vi "4Pi Objective Lock - EMBL.vi"(7 "Calling VI Ref":refnum<vi>) -> ()   [LabVIEW 2016]
uses:
  <vilib>/Utility/miscctls.llb/LVPointTypeDef.ctl
  4Pi Objective Lock Type Defs/4Pi Obj Lock - Notifier Type.ctl
  4Pi Objective Lock Type Defs/4Pi Obj Lock - Actions.ctl
  <vilib>/vision/Image Controls.llb/IMAQ Image.ctl
  4Pi Objective Lock Type Defs/4Pi Obj Lock - Lock Settings.ctl
  Hardware Configuration/Hardware Configuration Controls/Device Type.ctl
  Hardware Configuration/Hardware Configuration Controls/Device Function.ctl
  4Pi Objective Lock Type Defs/4Pi Obj Lock - Camera Settings.ctl
  Device Library/Cameras/Camera Controls/Generic Camera ROI.ctl
  Device Library/Cameras/Camera Controls/Generic Camera Actions.ctl
  Device Library/Stages/Stages Controls/Stage Actions.ctl
  <vilib>/addons/control/pid/pid.llb/PID (DBL Array).vi
  <vilib>/addons/control/pid/pid.llb/PID (DBL).vi
  <vilib>/addons/control/pid/NI_PID_pid.lvlib
  <vilib>/vision/NI_Vision_Development_Module.lvlib
panel:
  out "dxy (px)":dbl[](array[numeric])
  out "dz (µm)":dbl format="%.2f"
  in  "Main Tab":T1(tab)
  out "Z Move":bool
  out "XY Move":bool
  out "Measured X Position (px)":dbl=1.0 format="%.3g"
  out "Measured Y Position (px)":dbl=1.0 format="%.3g"
  out "Measured sx/sy":dbl=1.0 format="%.3g"
  out "Target X Position (px)":dbl=1.0 format="%.3g"
  out "Target Y Position (px)":dbl=1.0 format="%.3g"
  out "Target sx/sy":dbl=1.0 format="%.3g"
  out "Z Axis Position (µm)":dbl=1.0 format="%.4g"
  out "Y Axis Position (µm)":dbl=1.0 format="%.2g"
  out "X Axis Position (µm)":dbl=1.0 format="%.2g"
  out "Z Target and Fit Value (µm)":T2(graph)
  in  "Start Lock":bool
  out "Y Target and Fit Position (µm)":T2(graph)
  out "X Target and Fit Position (µm)":T2(graph)
  in  "Restart Lock":bool
  out "Fit Error":bool
  out "Move Limit Error":bool
  out "Target Z (µm)":dbl=1.0 format="%.3g"
  out "Measured Z (µm)":dbl=1.0 format="%.3g"
  out "Target X Position cc (px)":dbl=1.0 format="%.3g"
  out "Measured X Position cc (px)":dbl=1.0 format="%.3g"
  out "Measured Y Position cc (px)":dbl=1.0 format="%.3g"
  out "Target Y Position cc (px)":dbl=1.0 format="%.3g"
  in  "pixel size (µm)":dbl=0.01
  in  "X Update Scale Factor":dbl=0.01
  in  "Y Update Scale Factor":dbl=0.01
  in  "Z Update Scale Factor":dbl=0.2
  in  "Sample Z Step No.":u32=2
  in  "Sample Z Step Size (µm)":dbl=2.0
  in  "Update Delay (ms)":i32=10
  in  "D (Derivative)":dbl
  in  "I (Integral)":dbl
  in  "P (Proportional)":dbl=2.0
  in  "Invert Z Axis":bool
  in  "XY Drift Threshold":dbl=0.05
  in  "Abort If Error":bool
  in  "Flip XY Axis":bool
  in  "Invert X Axis":bool=TRUE
  in  "Invert Y Axis":bool=TRUE
  in  "Z Stage Move Limit (µm)":dbl=5.0
  in  "Z Drift Threshold":dbl=0.05
  in  "XY Stage Move Limit (µm)":dbl=1.0
  in  "Frame Accumulations":u16=10
  in  "XY Correction Active":bool=TRUE
  in  "Z Correction Active":bool=TRUE
  in  "Set Camera ROI":bool
  in  "Save Lock Settings":bool
  in  "Quit":bool
  # "Z Drift Settings"
  # "Camera Setup"
  # "XY Drift Settings"
  # "PID Control Values"
  # "General Settings"
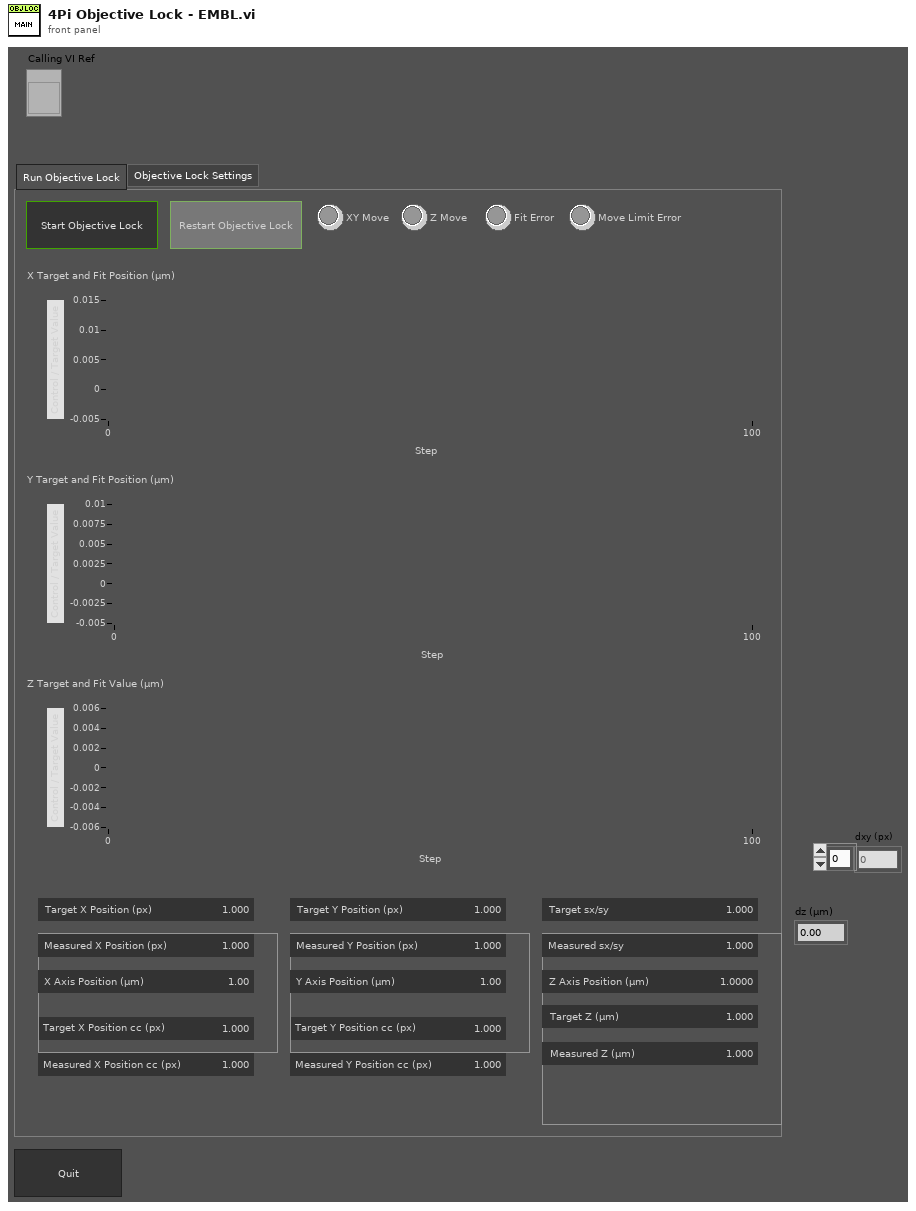
[diagram p1: front panel]
types:
  T1 = enum32{"Run Objective Lock", "Objective Lock Settings"}
  T2 = cluster{"Target 01":dbl, dbl, dbl, "Current 01":dbl, "Stage Pos":dbl}
  T3 = typedef "4Pi Obj Lock - Camera Settings.ctl" = cluster{"Exposure Time (s)":dbl, "H Offset":u16, "V Offset":u16, "H Width":u16, "V Width":u16}
  T4 = typedef "Device Function.ctl" = enum16{"Primary", "Secondary", "Overview", "Wide Field Drift Correction", "642 nm Excitation", "560 nm Excitation", "940 nm Excitation", "546 nm Excitation", "488 nm Excitation", "405 nm Excitation", "Objective Drift Correction", "4Pi Focus Lock", "4Pi Objective Lock", "Objective XY", "Objective Z", "Sample XY", "Sample Coarse Z", "Sample Z", "4Pi Lower", "4Pi Upper", "Mojo", "Adj Cavity", "Line Scanning", "Alert"}
  T5 = typedef "Device Type.ctl" = enum16{"AOTF", "Camera", "Deformable Mirror", "Laser", "Shutter", "Stage", "Waveform", "FPGA", "Email"}
  T6 = typedef "4Pi Obj Lock - Actions.ctl" = enum16{"Idle", "Start Lock", "Restart Lock", "Get Initial Position", "Get Target Z Position", "Get Ref Stack", "Cal Ref FFT", "Move To Init Z", "Get Current Z Position", "Get Current XY Position", "Get Current Position", "Check Drift", "Check Drift cc", "Move XYZ", "Move XY", "Move Z", "Update Plots", "Delay", "Abort", "Exit Loop", "Quit"}
  T7 = typedef "4Pi Obj Lock - Lock Settings.ctl" = cluster{"Z Drift Threshold":dbl, "Z Stage Move Limit (µm)":dbl, "XY Drift Threshold":dbl, "XY Stage Move Limit (µm)":dbl, "Frame Accumulations":u16, "Abort If Error":bool, "Flip XY Axis":bool, "Invert X Axis":bool, "Invert Y Axis":bool, "Invert Z Axis":bool, "Z Correction Active":bool, "XY Correction Active":bool, "PID Values":dbl[], "Update Delay (ms)":i32, "Sample Z Step Size (µm)":dbl, "Sample Z Step No.":u32, "Z Update Scale Factor":dbl, "Y Update Scale Factor":dbl, "X Update Scale Factor":dbl}
  T8 = typedef "4Pi Obj Lock - Notifier Type.ctl" = cluster{"Actions":T6, "Z Drift Threshold":dbl, "Z Stage Move Limit (µm)":dbl, "XY Drift Threshold":dbl, "XY Stage Move Limit (µm)":dbl, "Frame Accumulations":u16, "Abort If Error":bool, "Z Correction Active":bool, "XY Correction Active":bool, "PID Values":dbl[], "Running?":bool, "Update Delay (ms)":i32, "Cur Image (SGL)":T9, "Ref Stack (SGL)":T9[], "Sample Z (µm)":dbl[], "Initial Z Position (µm)":dbl, "Z Step Size (µm)":dbl, "Z Step No.":u32, "Ref FFT Stack (CSG)":T9[], "CC Image (SGL) ":T9, "Tmp Image FFT (CSG)":T9[], "CC Image Max (SGL)":T9}
  T9 = typedef "IMAQ Image.ctl" = refnum<image>
  T10 = enum16{"Always On", "Always Off", "Off While Running"}
  T11 = typedef "LVPointTypeDef.ctl" = cluster{"Horizontal":i16, "Vertical":i16}
  T12 = typedef "Image Type" = u32
  T13 = typedef "Generic Camera Actions.ctl" = enum16{"Status", "Live Preview", "Capture", "Abort", "Set Exposure Time (s)", "Get Exposure Time (s)", "Record Settings", "Set ROI", "Get ROI", "Defect Correction On/Off", "Cooler On/Off", "Fan On/Off", "Quit"}
  T14 = typedef "Generic Camera ROI.ctl" = cluster{"H_Offset":u16, "V_Offset":u16, "H_Width":u16, "V_Width":u16}
  T15 = typedef "Stage Actions.ctl" = enum16{"Get Position", "MVR", "MOVE", "HALT", "ONTARGET", "ERROR", "REFERENCE", "INIT", "VELOCITY", "STATUS", "EXIT", "HOME", "ZEROPOS", "NANOPOS", "ANALOG", "QUIT"}
  T16 = enum32{"Invalid", "Standard", "Closed", "Hidden", "Minimized", "Maximized"}
  T17 = cluster{"Target 01":dbl, dbl, dbl, "Current 01":dbl, "Stage Pos":dbl}[]
  T18 = typedef "Stage Status.ctl" = enum16{"Error", "Abort", "Busy", "On Target"}
  T19 = typedef "2D Gaussian - Best Fit Parameters.ctl" = cluster{"Amplitude":dbl, "X Position":dbl, "Y Position":dbl, "X Width":dbl, "Y Width":dbl, "Offset":dbl}
  T20 = cluster{"PID Values[0]":dbl, "PID Values[1]":dbl, "PID Values[2]":dbl}
  T21 = cluster{"PID Values[0]":dbl, "PID Values[1]":dbl, "PID Values[2]":dbl}[]
  T22 = typedef "LVRectTypeDef.ctl" = cluster{"Left":i16, "Top":i16, "Right":i16, "Bottom":i16}
  T23 = typedef "LVBoundsTypeDef.ctl" = cluster{"Width":u32, "Height":u32}
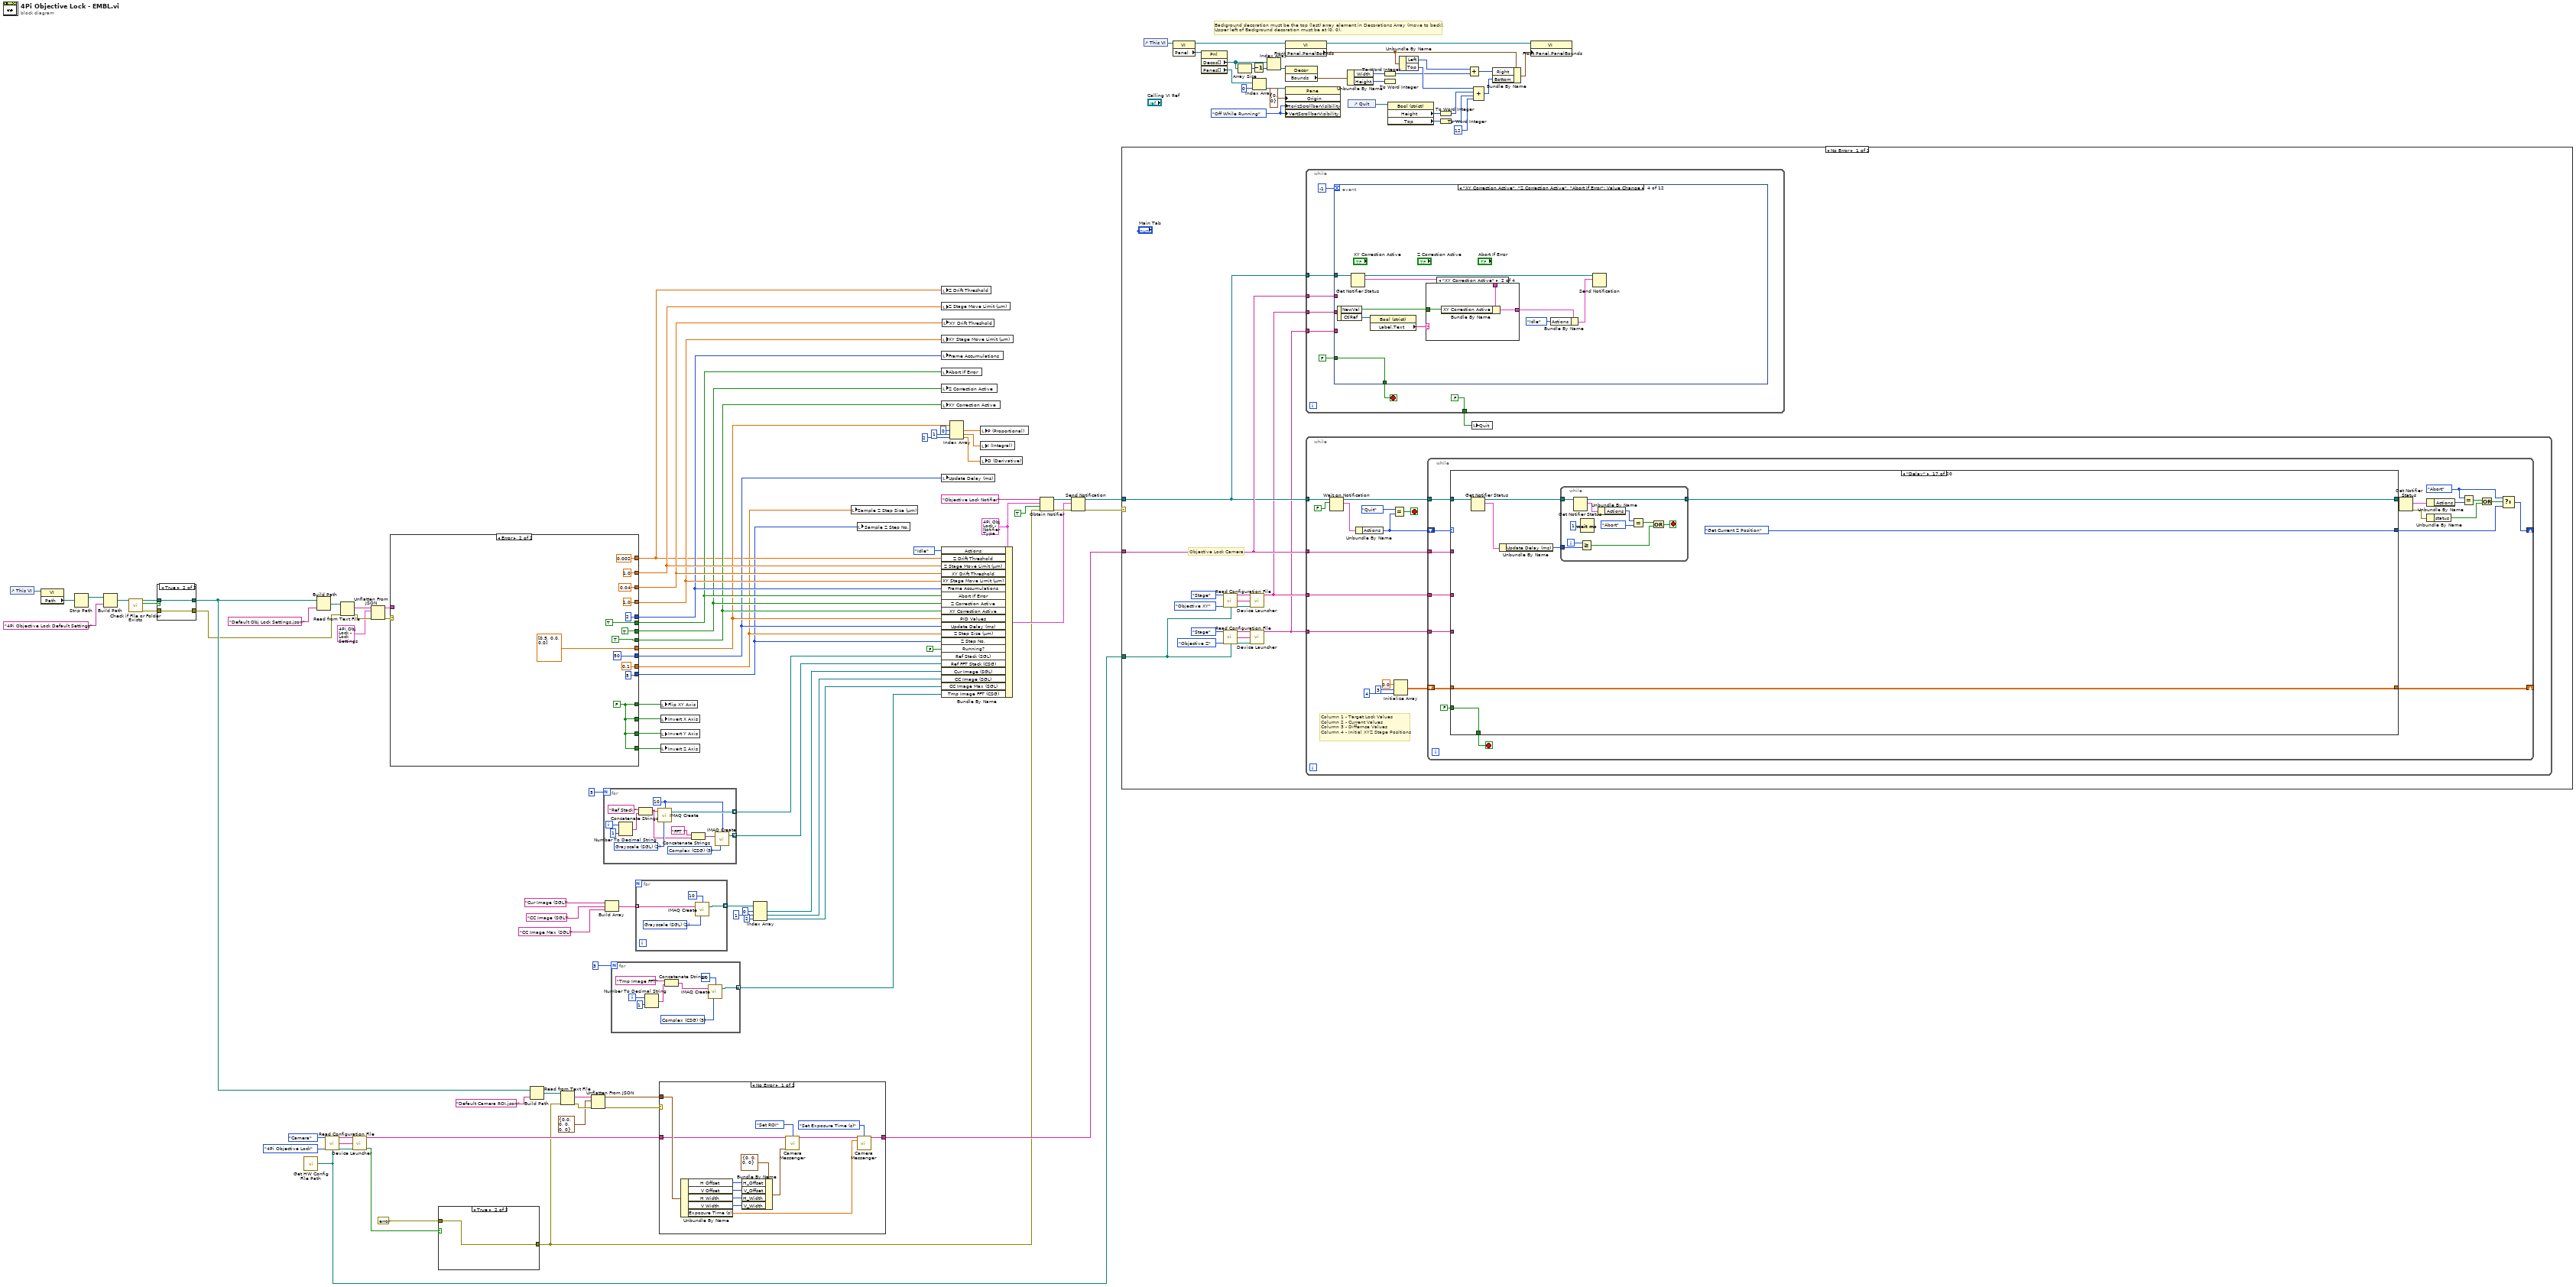
[diagram p0: block diagram]
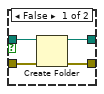
[diagram p2: hidden frame]
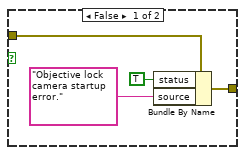
[diagram p3: hidden frame]
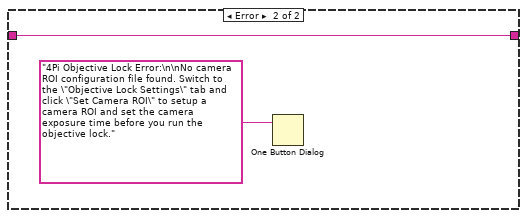
[diagram p4: hidden frame]
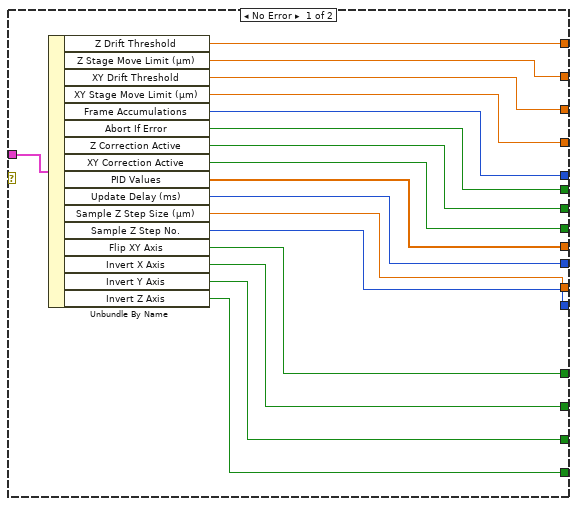
[diagram p5: hidden frame]
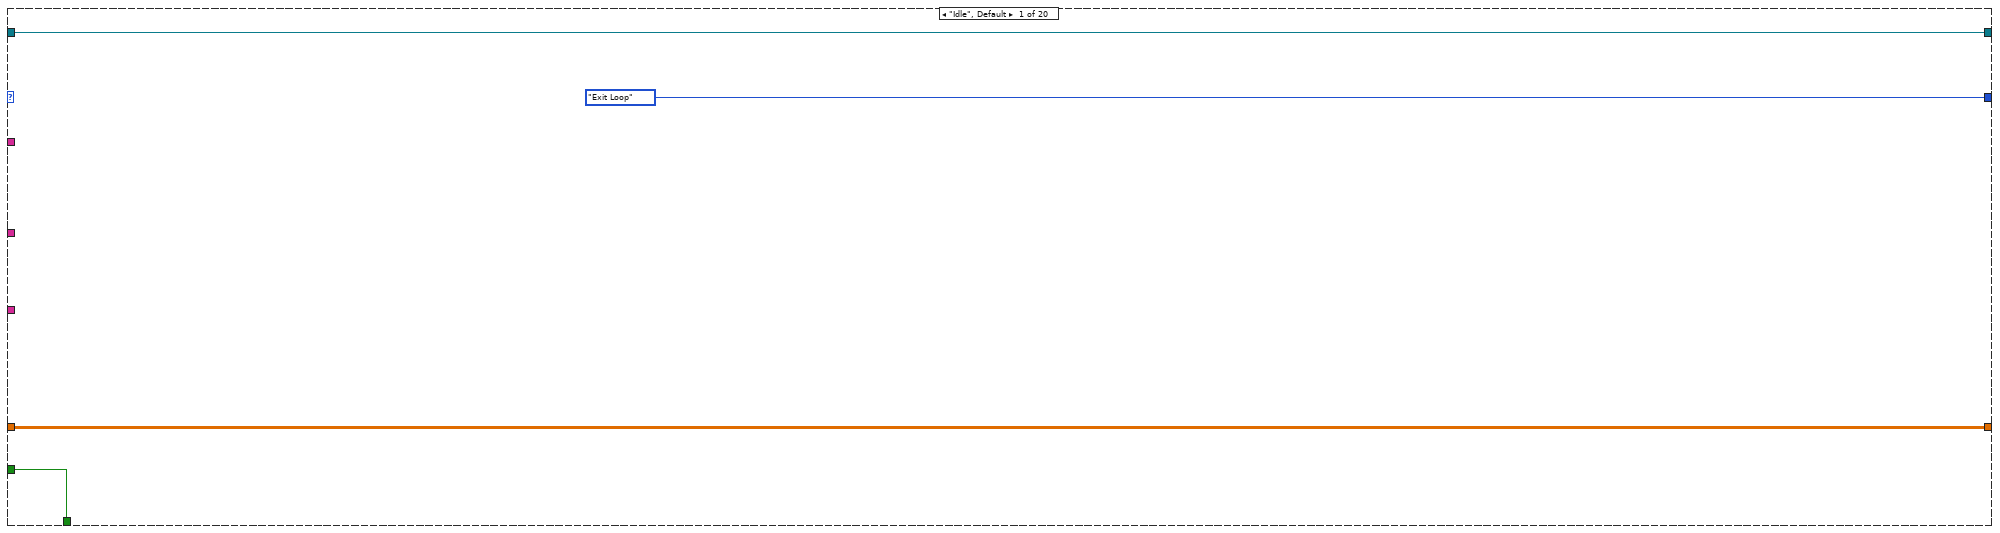
[diagram p6: hidden frame]
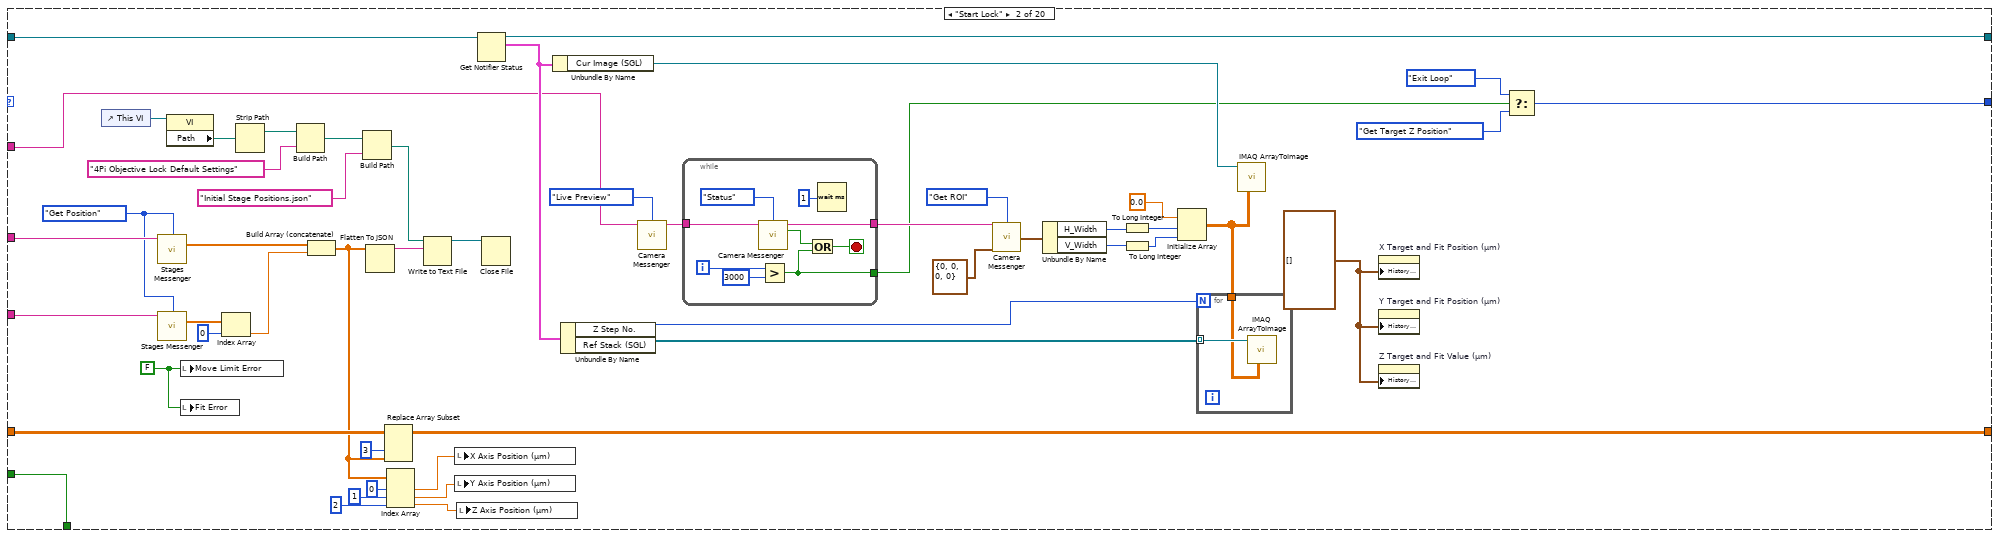
[diagram p7: hidden frame]
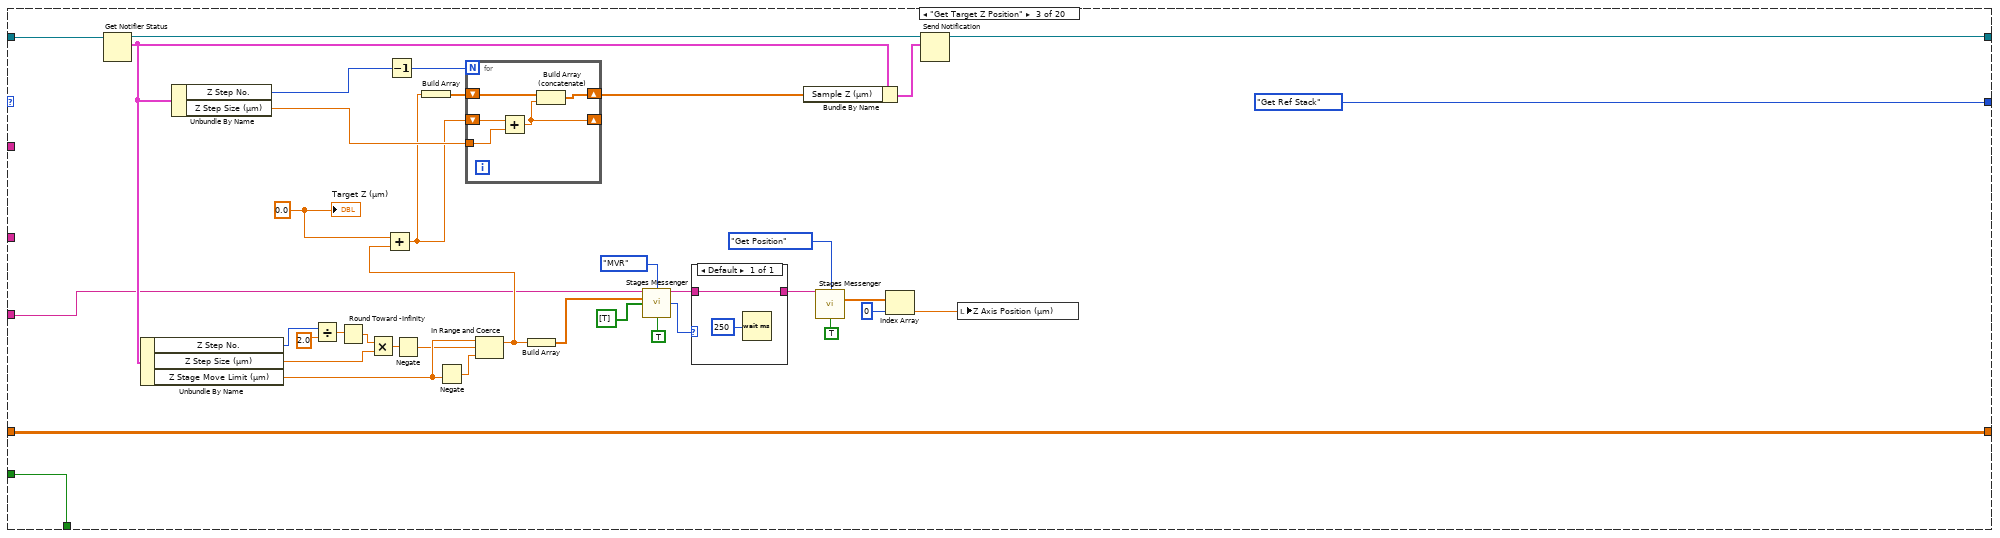
[diagram p8: hidden frame]
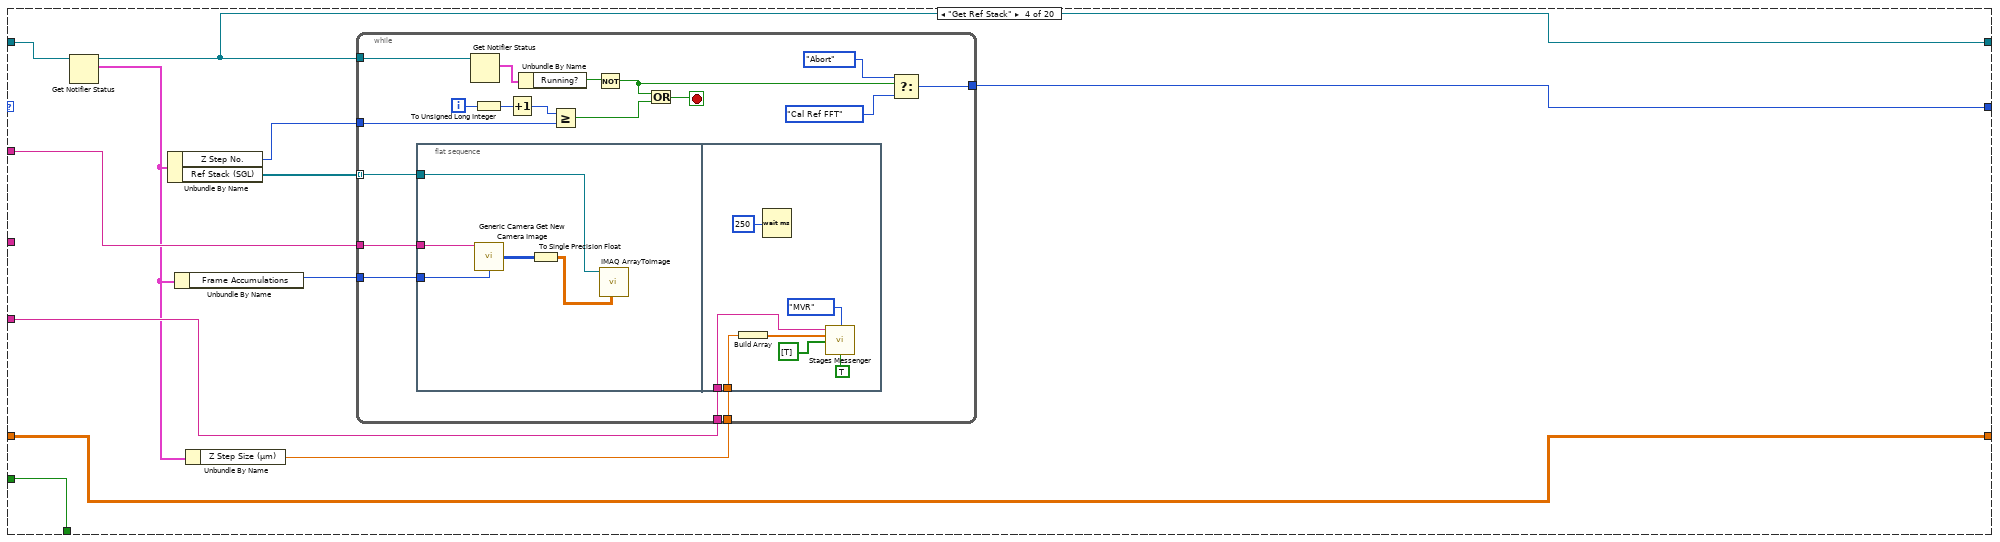
[diagram p9: hidden frame]
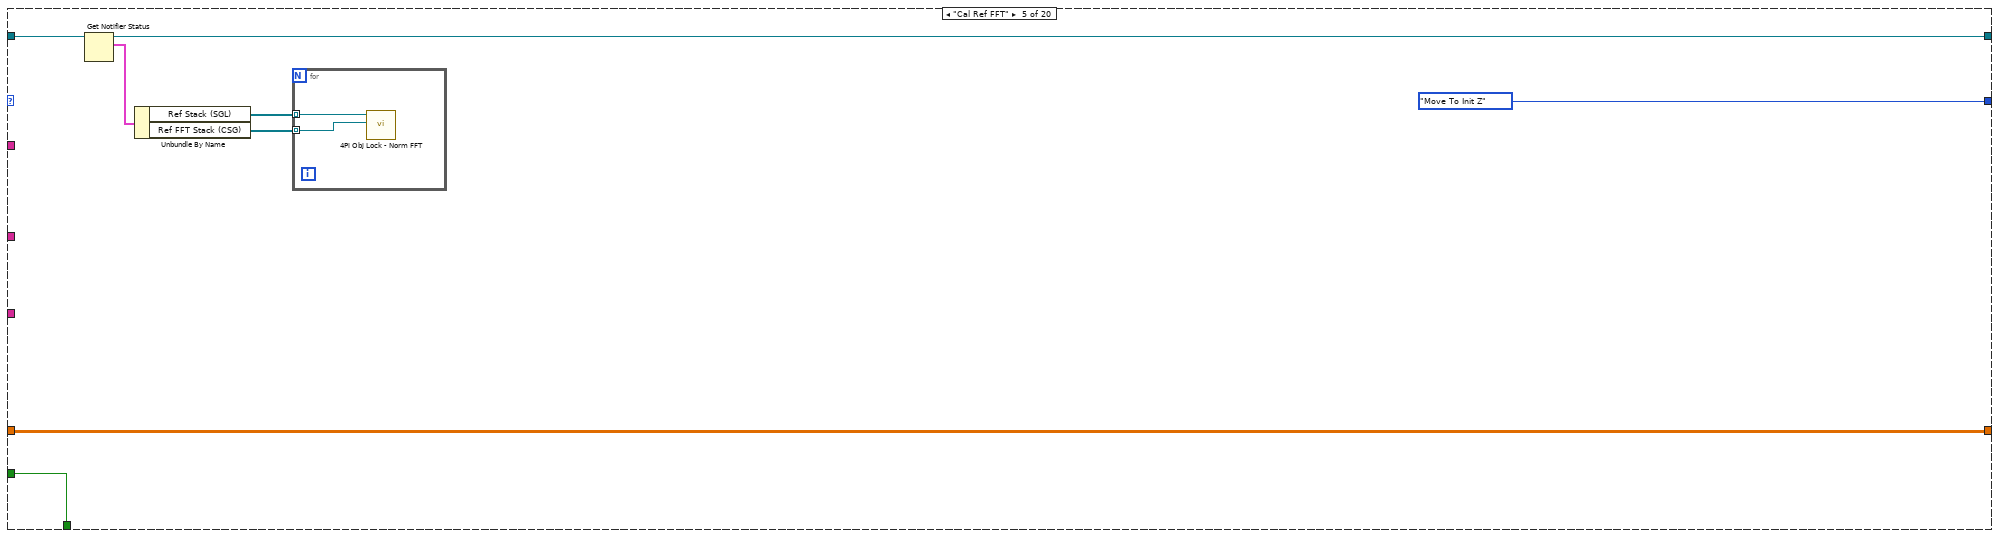
[diagram p10: hidden frame]
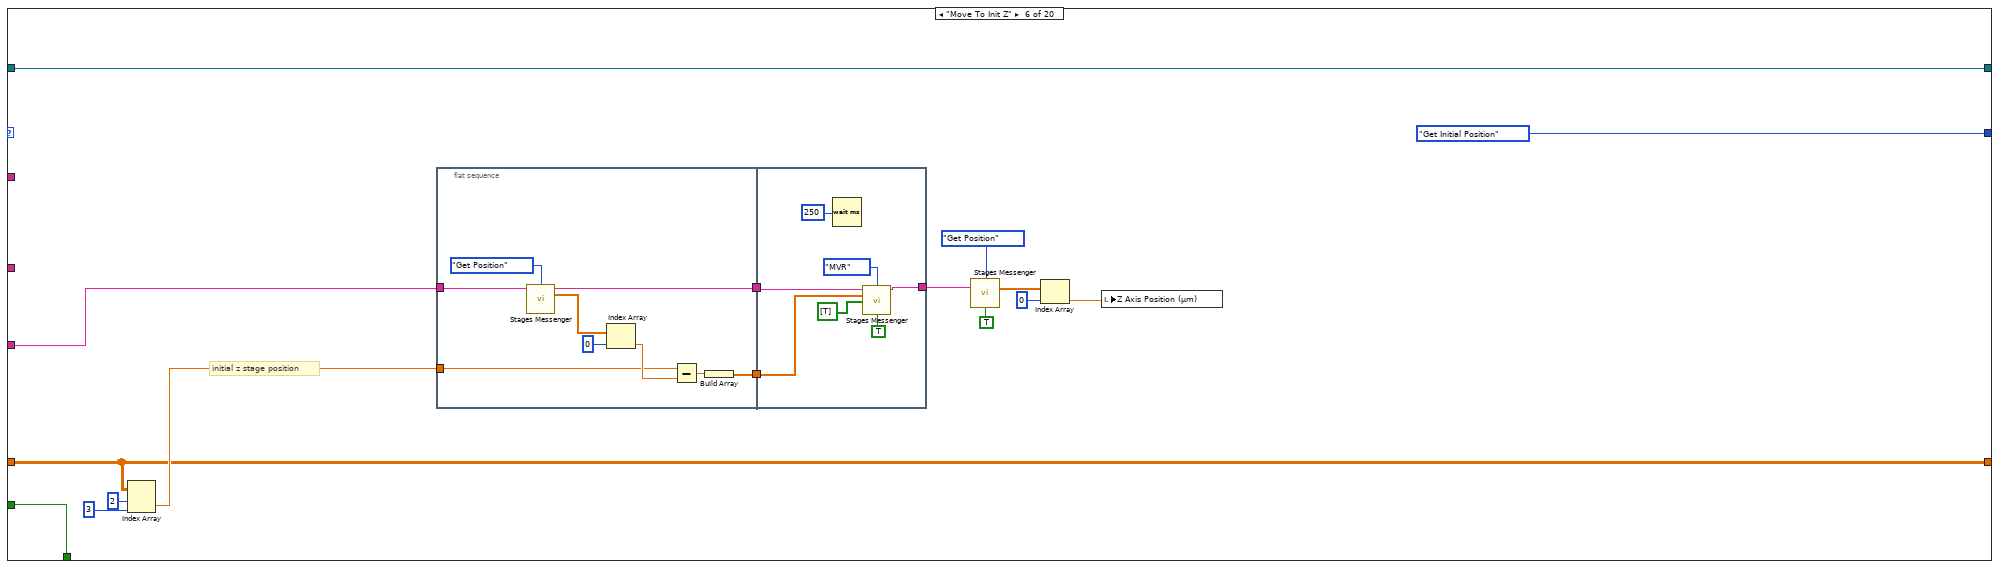
[diagram p11: hidden frame]
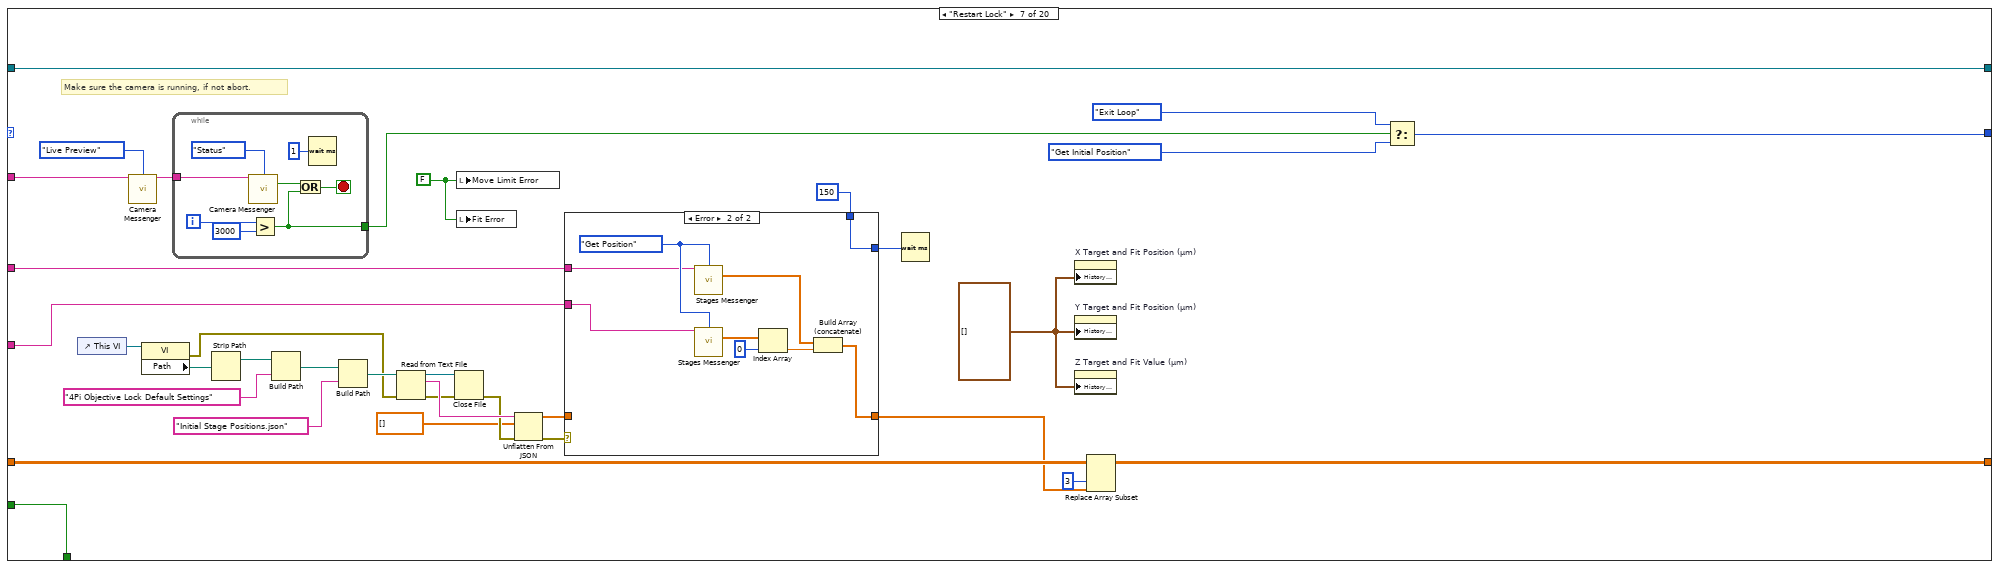
[diagram p12: hidden frame]
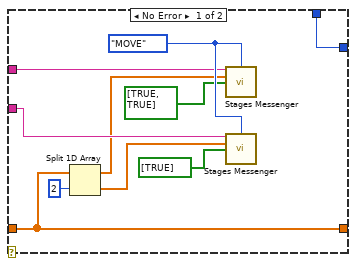
[diagram p13: hidden frame]
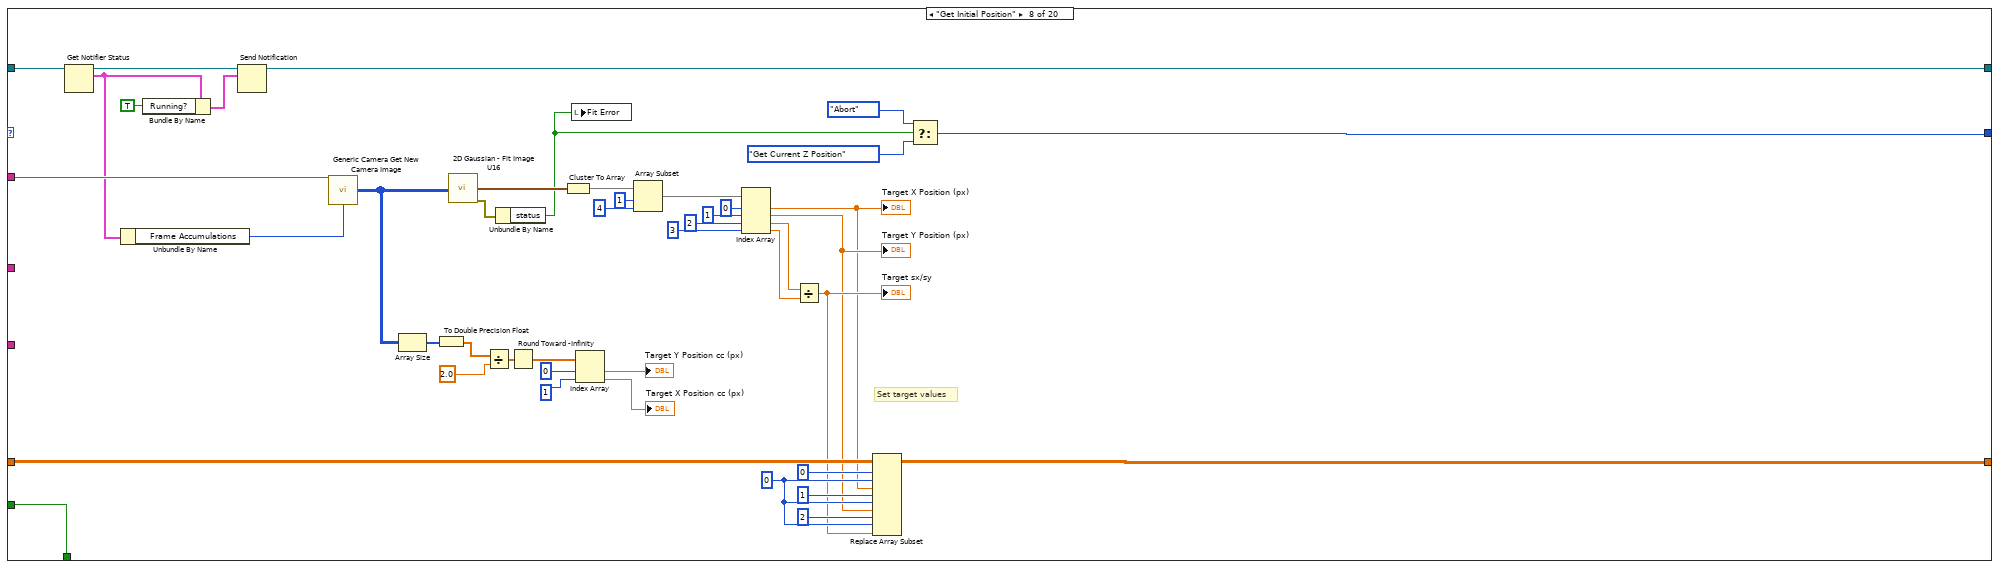
[diagram p14: hidden frame]
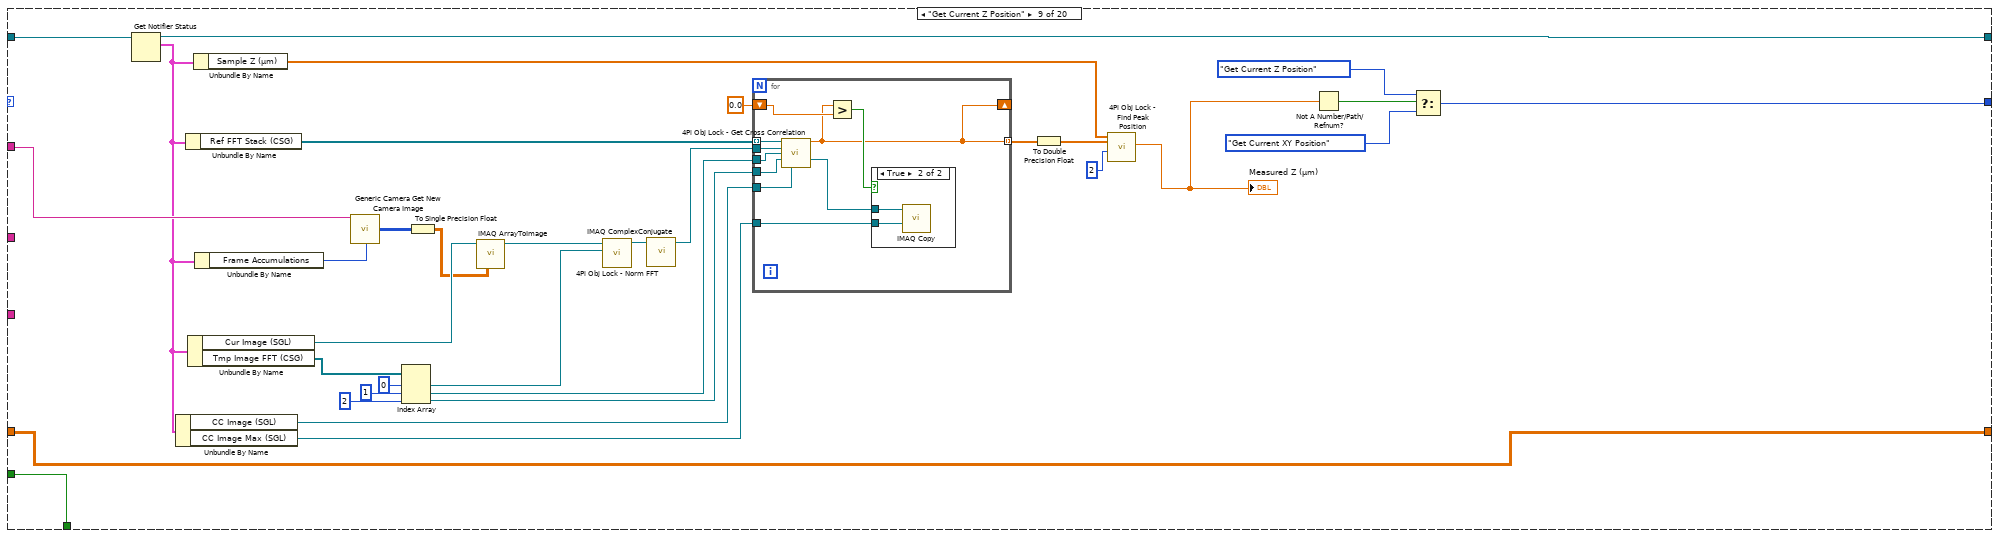
[diagram p15: hidden frame]
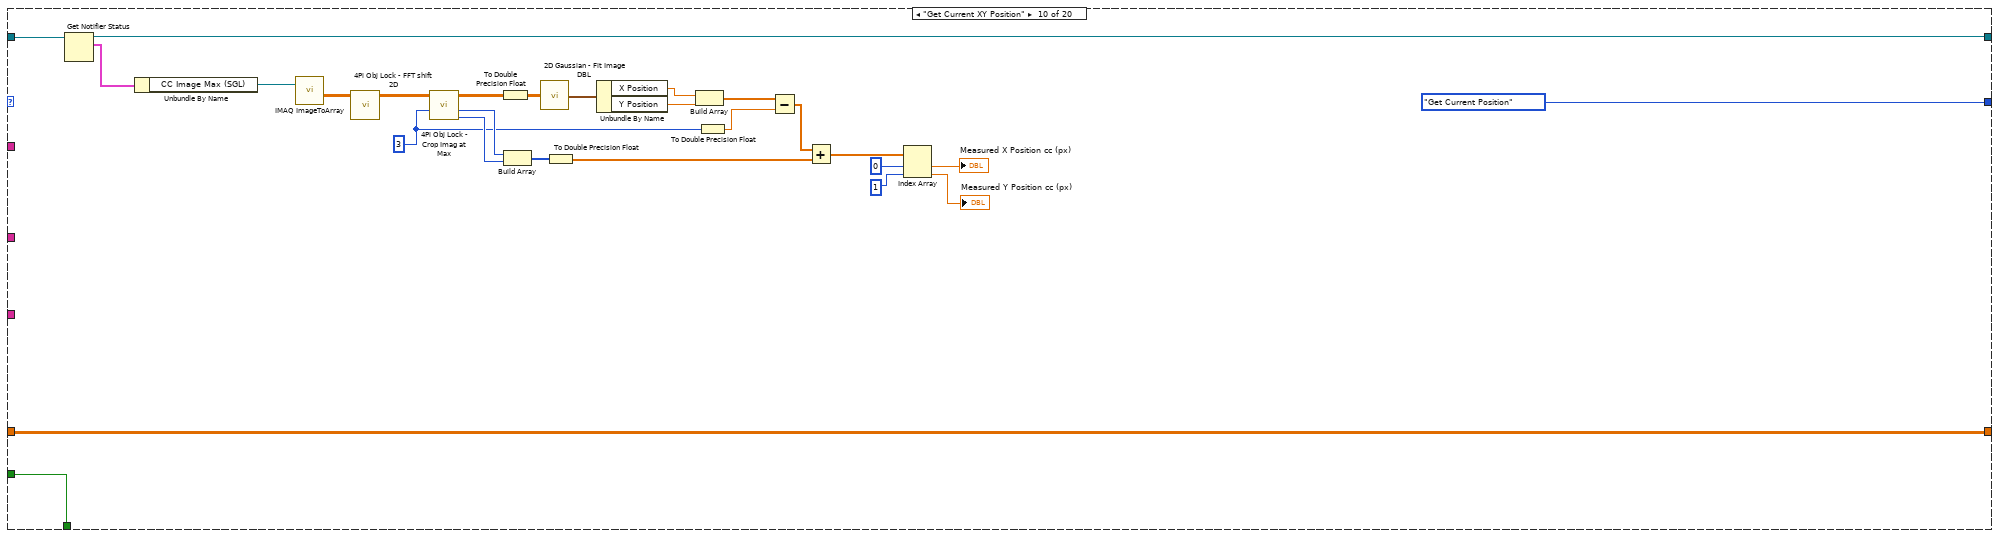
[diagram p17: hidden frame]
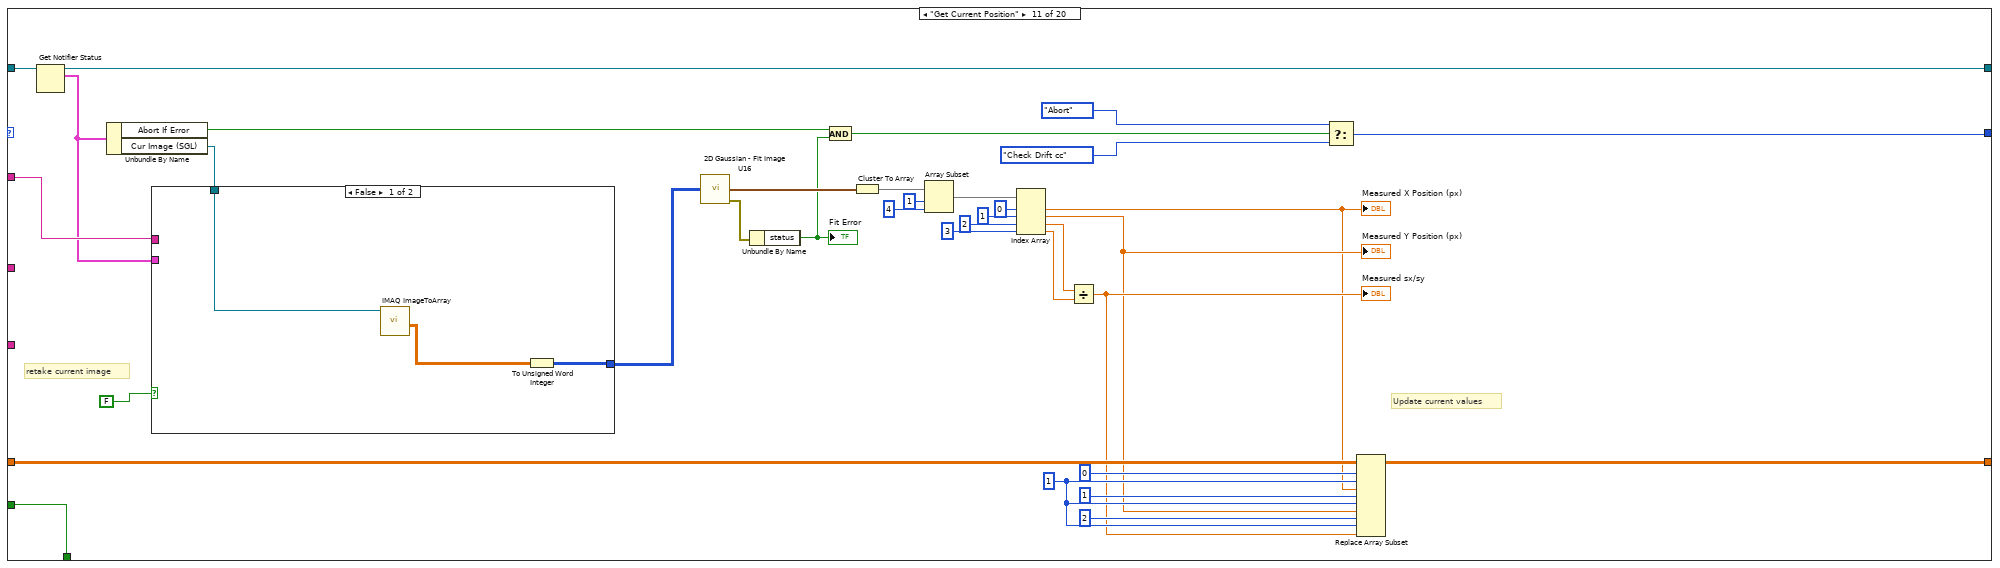
[diagram p18: hidden frame]
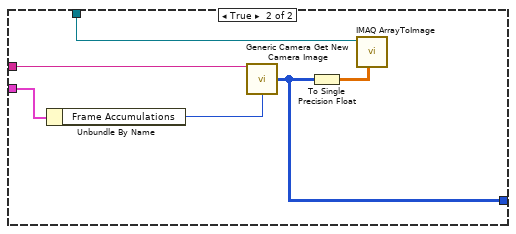
[diagram p19: hidden frame]
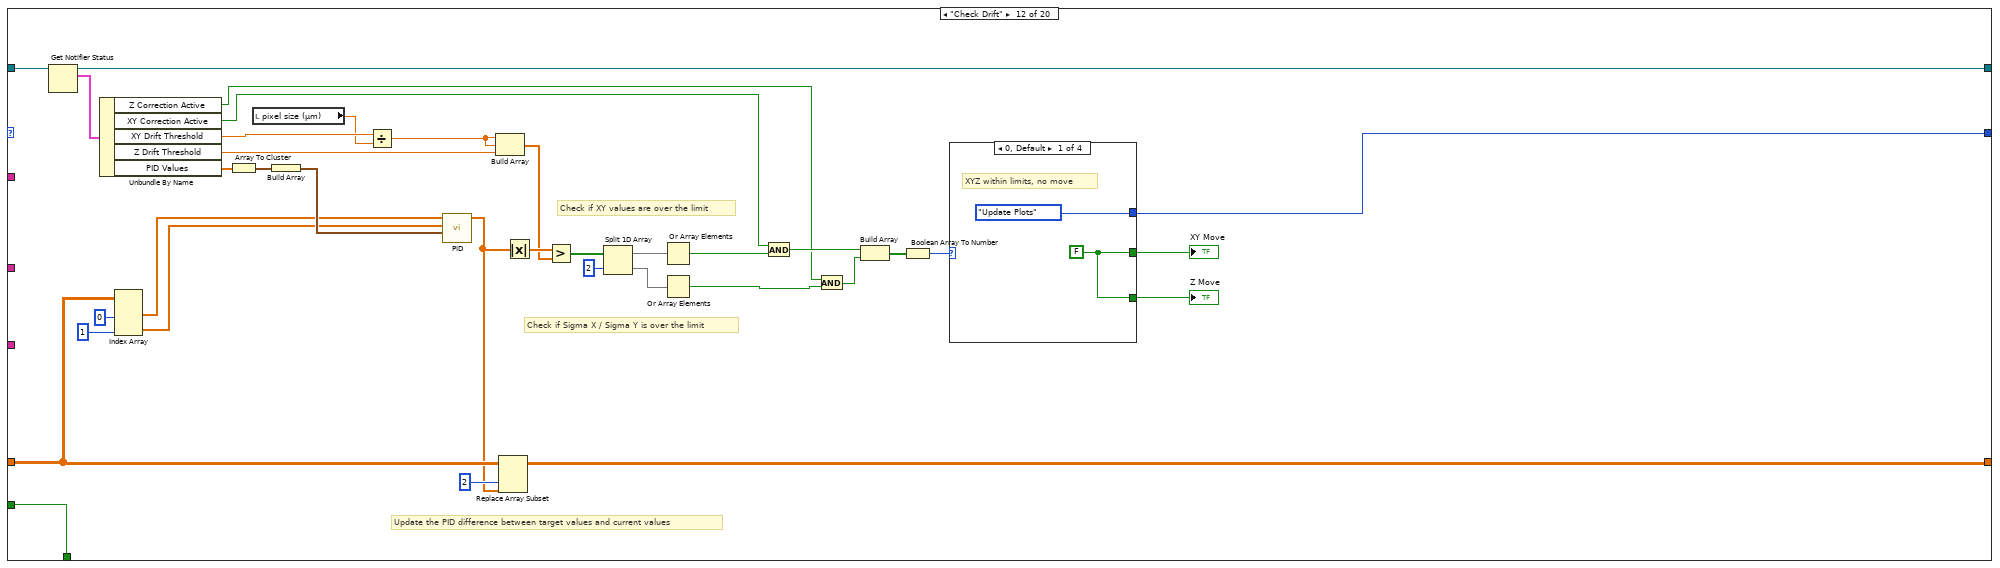
[diagram p20: hidden frame]
diagram:
  w78 = T8 {"Actions"=enum."Idle", "Z Drift Threshold"=0.05, "Z Stage Move Limit (µm)"=1.0, "XY Drift Threshold"=0.05, "XY Stage Move Limit (µm)"=1.0, "Frame Accumulations"=10, "Abort If Error"=FALSE, "Z Correction Active"=FALSE, "XY Correction Active"=FALSE, "PID Values"=[], "Running?"=FALSE, "Update Delay (ms)"=0, "Cur Image (SGL)"=refnum, "Ref Stack (SGL)"=[], "Sample Z (µm)"=[], "Initial Z Position (µm)"=0.0, "Z Step Size (µm)"=2.0, "Z Step No."=2, "Ref FFT Stack (CSG)"=[], "CC Image (SGL) "=refnum, "Tmp Image FFT (CSG)"=[], "CC Image Max (SGL)"=refnum} ("4Pi Obj Lock")
  w95 = T10."Off While Running" ("Vertical Scrollbar Visibility")
  # "Background decoration must be the top (last) array element in Decorations Array (move to back).\nUpper left of Background decoration must be at (0, 0)."
  n1 = control-ref of="This VI"() -> (w66:refnum<vi>)
  n2 = property class="VI"(reference=w66) -> ("Path"=w48:path)  [unwired: 1 in, 2 out]
  n3 = Strip Path(path=w48) -> (stripped path=w47:path)  [unwired: 1 out]
  n4 = Build Path(base path=w47, name or relative path="4Pi Objective Lock Default Settings") -> (appended path=w24:path)
  n5 = call <vilib>:"Check if File or Folder Exists.vi"("path"=w24) -> ("error out"=w20:errorcluster, "file or folder exists?"=w23:bool, "dup path"=w22:path)  [unwired: 8 in]
  n6 = case shown="True" w23 {
    tunnel: w22 -> [w116 w118]
    tunnel: [w115 w118] -> w21
    tunnel: w20 -> [w114 w117]
    tunnel: [w113 w117] -> w19
    frame False {
      n7 = Create Folder(path (use dialog)=w116, error in=w114) -> (created path=w115:path, error out=w113:errorcluster)  [unwired: 1 in, 1 out]
    }
    frame True {
    }
  }
  n8 = call "Get HW Config File Path.vi"() -> ("File Path"=w56:path)  [unwired: 14 in, 1 out]
  n9 = Build Path(base path=w21, name or relative path="Default Obj Lock Settings.json") -> (appended path=w75:path)
  n10 = call "Read Configuration File.vi"("Device Type"=Device_Type."Camera", "Device Function"=Device_Function."4Pi Objective Lock", "Config File Path"=w56) -> ("Unique Notifier Name"=w63:string, "Device Ports/IDs/Channels"=w65:string[], "Device Engine Path"=w64:path)  [unwired: 9 in, 1 out]
  n11 = Read from Text File(file (use dialog)=w75, error in=w19) -> (text=w74:string, error out=w73:errorcluster)  [unwired: 2 in, 2 out]
  n12 = call "Device Launcher.vi"("Notifier Name"=w63, "Device Ports/IDs/Channels"=w65, "Device Engine Path"=w64) -> ("Notifier Name"=w54:string, "Running?"=w60:bool)  [unwired: 11 in]
  n13 = Unflatten From JSON(JSON string=w74, type and defaults=T7 {"Z Drift Threshold"=0.05, "Z Stage Move Limit (µm)"=1.0, "XY Drift Threshold"=0.05, "XY Stage Move Limit (µm)"=1.0, "Frame Accumulations"=10, "Abort If Error"=FALSE, "Flip XY Axis"=FALSE, "Invert X Axis"=FALSE, "Invert Y Axis"=FALSE, "Invert Z Axis"=FALSE, "Z Correction Active"=TRUE, "XY Correction Active"=TRUE, "PID Values"=[], "Update Delay (ms)"=0, "Sample Z Step Size (µm)"=2.0, "Sample Z Step No."=2, "Z Update Scale Factor"=2.0, "Y Update Scale Factor"=2.0, "X Update Scale Factor"=2.0} ("Lock Settings"), error in (no error)=w73) -> (value=w70:T7, error out=w71:errorcluster)  [unwired: 4 in]
  n14 = case shown="Error" w71 {
    tunnel: [w134 0.002 ("Z Drift Threshold")] -> w25
    tunnel: [w133 1.0 ("Z Stage Move Limit (µm)")] -> w40
    tunnel: [w131 0.04 ("XY Drift Threshold")] -> w39
    tunnel: [w132 1.0 ("XY Stage Move Limit (µm)")] -> w38
    tunnel: [w130 u16 2 ("Frame Accumulations")] -> w37
    tunnel: [w129 TRUE ("Abort If Error")] -> w36
    tunnel: w70 -> [w135 _]
    tunnel: [w128 TRUE ("Z Correction Active")] -> w35
    tunnel: [w127 TRUE ("XY Correction Active")] -> w34
    tunnel: [w126 dbl[] [0.5, 0.0, 0.0] ("PID Values")] -> w33
    tunnel: [w125 u16 50 ("Update Delay (ms)")] -> w26
    tunnel: [w124 w138] -> w42
    tunnel: [w123 w138] -> w43
    tunnel: [w122 w138] -> w44
    tunnel: [w121 w138] -> w45
    tunnel: [w120 0.1 ("Sample Z Step Size (µm)")] -> w5
    tunnel: [w119 u32 5 ("Sample Z Step No.")] -> w4
    frame No Error {
      n15 = Unbundle By Name(w135) -> ("Z Drift Threshold"=w134:dbl, "Z Stage Move Limit (µm)"=w133:dbl, "XY Drift Threshold"=w131:dbl, "XY Stage Move Limit (µm)"=w132:dbl, "Frame Accumulations"=w130:u16, "Abort If Error"=w129:bool, "Z Correction Active"=w128:bool, "XY Correction Active"=w127:bool, "PID Values"=w126:dbl[], "Update Delay (ms)"=w125:i32, "Sample Z Step Size (µm)"=w120:dbl, "Sample Z Step No."=w119:u32, "Flip XY Axis"=w121:bool, "Invert X Axis"=w122:bool, "Invert Y Axis"=w123:bool, "Invert Z Axis"=w124:bool)
    }
    frame Error {
      w138 = FALSE ("Flip XY Axis")
    }
  }
  n16 = case shown="True" w60 {
    tunnel: errorcluster {"status"=FALSE, "code"=0, "source"=""} ("Error") -> [w152 w153]
    tunnel: [w149 w153] -> w46
    frame False {
      n17 = Bundle By Name(cluster=w152, "status"=TRUE, "source"="Objective lock camera startup error." ("name or relative path")) -> (w149:errorcluster)
    }
    frame True {
    }
  }
  n18 = Build Path(base path=w21, name or relative path="Default Camera ROI.json") -> (appended path=w50:path)
  n19 = Read from Text File(file (use dialog)=w50, error in=w46) -> (text=w68:string, error out=w67:errorcluster)  [unwired: 2 in, 2 out]
  n20 = Unflatten From JSON(JSON string=w68, type and defaults=T3 {"Exposure Time (s)"=0.0, "H Offset"=0, "V Offset"=0, "H Width"=0, "V Width"=0} ("Camera Settings"), error in (no error)=w67) -> (value=w53:T3, error out=w58:errorcluster)  [unwired: 4 in]
  n21 = for {
    N: 5 -> [_]
    tunnel: [w165] -> w17 mode=indexing
    tunnel: [w154] -> w16 mode=indexing
    i -> [w164]
    w159 = T12 3 items=["Grayscale (U8)", "Grayscale (I16)", "Grayscale (SGL)", "Complex (CSG)", "RGB (U32)", "HSL (U32)", "RGB (U64)", "Grayscale (U16)"] ("Image Type")
    w160 = T12 2 items=["Grayscale (U8)", "Grayscale (I16)", "Grayscale (SGL)", "Complex (CSG)", "RGB (U32)", "HSL (U32)", "RGB (U64)", "Grayscale (U16)"] ("Image Type")
    w156 = 10 ("Border Size")
    n22 = Number To Decimal String(number=w164, width (-)=i16 1) -> (decimal integer string=w162:string)
    n23 = Concatenate Strings("Ref Stack " ("string"), w162) -> (w155:string)
    n24 = call "IMAQ Create"("Border Size"=w156, "Image Name"=w155, "Image Type"=w160) -> ("New Image"=w165:T9)  [unwired: 2 in, 1 out]
    n25 = Concatenate Strings("FFT " ("string"), w155) -> (w158:string)
    n26 = call "IMAQ Create"("Border Size"=w156, "Image Name"=w158, "Image Type"=w159) -> ("New Image"=w154:T9)  [unwired: 2 in, 1 out]
  }
  n27 = Build Array("Cur Image (SGL)" ("Image Name"), "CC Image (SGL)" ("Image Name"), "CC Image Max (SGL)" ("Image Name")) -> (w11:string[])
  n28 = for {
    N: 3 -> [_]
    tunnel: [w171] -> w6 mode=indexing
    i -> [w167]
    w172 = T12 3 items=["Grayscale (U8)", "Grayscale (I16)", "Grayscale (SGL)", "Complex (CSG)", "RGB (U32)", "HSL (U32)", "RGB (U64)", "Grayscale (U16)"] ("Image Type")
    n29 = Number To Decimal String(number=w167, width (-)=i16 1) -> (decimal integer string=w170:string)
    n30 = Concatenate Strings("Tmp Image FFT" ("Image Name"), w170) -> (w166:string)
    n31 = call "IMAQ Create"("Border Size"=10, "Image Name"=w166, "Image Type"=w172) -> ("New Image"=w171:T9)  [unwired: 2 in, 1 out]
  }
  n32 = for {
    tunnel: w11 -> [w175] mode=indexing
    tunnel: [w174] -> w10 mode=indexing
    w176 = T12 2 items=["Grayscale (U8)", "Grayscale (I16)", "Grayscale (SGL)", "Complex (CSG)", "RGB (U32)", "HSL (U32)", "RGB (U64)", "Grayscale (U16)"] ("Image Type")
    n33 = call "IMAQ Create"("Border Size"=10, "Image Name"=w175, "Image Type"=w176) -> ("New Image"=w174:T9)  [unwired: 2 in, 1 out]
  }
  n34 = case shown="No Error" w58 {
    tunnel: w54 -> [w181 w192]
    tunnel: w53 -> [w190 _]
    tunnel: [w178 w192] -> w52
    frame No Error {
      n35 = Unbundle By Name(w190) -> ("H Offset"=w185:u16, "V Offset"=w186:u16, "H Width"=w187:u16, "V Width"=w188:u16, "Exposure Time (s)"=w180:dbl)
      n36 = Bundle By Name(cluster=T14 {"H_Offset"=0, "V_Offset"=0, "H_Width"=0, "V_Width"=0} ("General Camera ROI"), "H_Offset"=w185, "V_Offset"=w186, "H_Width"=w187, "V_Width"=w188) -> (w184:T14)
      n37 = call "Camera Messenger.vi"("Notifier Name"=w181, "General Camera Actions"=Generic_Camera_Actions."Set ROI", "Camera ROI"=w184) -> ("Notifier Name Dup"=w179:string)  [unwired: 7 in, 5 out]
      n38 = call "Camera Messenger.vi"("Notifier Name"=w179, "General Camera Actions"=Generic_Camera_Actions."Set Exposure Time (s)", "Exposure Time (s)"=w180) -> ("Notifier Name Dup"=w178:string)  [unwired: 7 in, 5 out]
    }
    frame Error {
      n39 = One Button Dialog(message="4Pi Objective Lock Error:\n\nNo camera ROI configuration file found. Switch to the \"Objective Lock Settings\" tab and click \"Set Camera ROI\" to setup a camera ROI and set the camera exposure time before you run the objective lock.") -> ()  [unwired: 1 in, 1 out]
    }
  }
  n40 = local write "Flip XY Axis"(w45) -> ()
  n41 = local write "Invert X Axis"(w44) -> ()
  n42 = local write "Invert Y Axis"(w43) -> ()
  n43 = local write "Invert Z Axis"(w42) -> ()
  n44 = Index Array(array=w10, index #1=0 ("index"), index #2=1 ("index"), index #3=2 ("index")) -> (element #1=w9:T9, element #2=w8:T9, element #3=w1:T9)
  n45 = local write "Sample Z Step Size (µm)"(w5) -> ()
  n46 = local write "Sample Z Step No."(w4) -> ()
  n47 = Bundle By Name(cluster=w78, "Actions"=4Pi_Obj_Lock_-_Actions."Idle", "Z Drift Threshold"=w25, "Z Stage Move Limit (µm)"=w40, "XY Drift Threshold"=w39, "XY Stage Move Limit (µm)"=w38, "Frame Accumulations"=w37, "Abort If Error"=w36, "Z Correction Active"=w35, "XY Correction Active"=w34, "PID Values"=w33, "Update Delay (ms)"=w26, "Z Step Size (µm)"=w5, "Z Step No."=w4, "Running?"=FALSE ("Obj Lock Active?"), "Ref Stack (SGL)"=w17, "Ref FFT Stack (CSG)"=w16, "Cur Image (SGL)"=w9, "CC Image (SGL)"=w8, "CC Image Max (SGL)"=w1, "Tmp Image FFT (CSG)"=w6) -> (w77:T8)
  n48 = local write "Z Drift Threshold"(w25) -> ()
  n49 = local write "Z Stage Move Limit (µm)"(w40) -> ()
  n50 = local write "XY Stage Move Limit (µm)"(w38) -> ()
  n51 = local write "Frame Accumulations"(w37) -> ()
  n52 = local write "Abort If Error"(w36) -> ()
  n53 = local write "Z Correction Active"(w35) -> ()
  n54 = local write "XY Correction Active"(w34) -> ()
  n55 = local write "Update Delay (ms)"(w26) -> ()
  n56 = local write "XY Drift Threshold"(w39) -> ()
  n57 = Index Array(array=w33, index #1=0 ("index"), index #2=1 ("index"), index #3=2 ("index")) -> (element #1=w29:dbl, element #2=w27:dbl, element #3=w28:dbl)
  n58 = local write "P (Proportional)"(w29) -> ()
  n59 = local write "I (Integral)"(w27) -> ()
  n60 = local write "D (Derivative)"(w28) -> ()
  n61 = Obtain Notifier(name (unnamed)="Objective Lock Notifier", notification data type=w78, create if not found? (T)=TRUE, error in (no error)=w46) -> (notifier out=w80:refnum<notifier>, error out=w81:errorcluster)  [unwired: 1 out]
  n62 = Send Notification(notification=w77, notifier=w80, error in (no error)=w81) -> (notifier out=w79:refnum<notifier>, error out=w57:errorcluster)
  n63 = case shown="No Error" w57 {
    tunnel: w56 -> [w197 _]
    tunnel: w79 -> [w195 _]
    tunnel: w52 -> [w196 _]
    frame No Error {
      # "Objective Lock Camera"
      n64 = call "Read Configuration File.vi"("Device Type"=Device_Type."Stage", "Device Function"=Device_Function."Objective XY", "Config File Path"=w197) -> ("Unique Notifier Name"=w205:string, "Device Ports/IDs/Channels"=w203:string[], "Device Engine Path"=w204:path)  [unwired: 9 in, 1 out]
      n65 = call "Read Configuration File.vi"("Device Type"=Device_Type."Stage", "Device Function"=Device_Function."Objective Z", "Config File Path"=w197) -> ("Unique Notifier Name"=w200:string, "Device Ports/IDs/Channels"=w202:string[], "Device Engine Path"=w201:path)  [unwired: 9 in, 1 out]
      n66 = call "Device Launcher.vi"("Notifier Name"=w205, "Device Ports/IDs/Channels"=w203, "Device Engine Path"=w204) -> ("Notifier Name"=w194:string)  [unwired: 11 in, 1 out]
      n67 = call "Device Launcher.vi"("Notifier Name"=w200, "Device Ports/IDs/Channels"=w202, "Device Engine Path"=w201) -> ("Notifier Name"=w193:string)  [unwired: 11 in, 1 out]
      n68 = while {
        tunnel: [FALSE] -> w208
        tunnel: w196 -> [w995]
        tunnel: w195 -> [w994]
        tunnel: w194 -> [w993]
        tunnel: w193 -> [w992]
        stop <- w997 stop-if-true
        n69 = event shown="[3] \"XY Correction Active\", \"Z Correction Active\", \"Abort If Error\": Value Change" {
          selector: _ -> [_ _ _ _ _ _ _ _ _ _ _ _]
          dyn-events: _ -> [_ _ _ _ _ _ _ _ _ _ _ _]
          timeout: -1 -> [_ _ _ _ _ _ _ _ _ _ _ _]
          tunnel: FALSE -> [w1000 w1004 w1007 w1017 w1037 w1072 w1099 w1106 w1135 w1145 w1152 _]
          tunnel: [w1000 w1004 w1007 w1017 w1037 w1072 w1099 w1106 w1135 w1145 w1152 w1162] -> w997
          tunnel: w995 -> [_ _ w1006 _ _ _ _ _ _ _ _ _]
          tunnel: w994 -> [_ _ _ w1016 w1034 w1075 w1098 w1105 w1134 w1144 w1151 w1157]
          tunnel: w993 -> [_ _ _ _ _ _ _ _ _ _ _ _]
          tunnel: w992 -> [_ _ _ _ _ _ _ _ _ _ _ _]
          event Timeout {
            n70 = event-data() -> ()  [unwired: 1 in, 1 out]
          }
          event Application Instance Close? {
            n71 = event-data() -> ()  [unwired: 1 in, 1 out]
            n72 = control-ref of="This VI"() -> (w1001:refnum<vi>)
            n73 = invoke class="VI" method="FP.Open"(reference=w1001, "Activate"=TRUE ("Activate?"), "State"=T16."Standard") -> ()  [unwired: 2 in, 5 out]
            n74 = event-data("Discard?"=TRUE) -> ()  [unwired: 1 in, 1 out]
          }
          event "Set Camera ROI": Value Change {
            n75 = event-data() -> ()  [unwired: 1 in, 2 out]
            n76 = call "4Pi Obj Lock - Setup Camera.vi"("Camera Notifier Name"=w1006) -> ()  [unwired: 14 in, 1 out]
          }
          event "XY Correction Active", "Z Correction Active", "Abort If Error": Value Change {
            n77 = event-data() -> ("NewVal"=w1012:bool, "CtlRef"=w1015:refnum<vi>)  [unwired: 1 in]
            n78 = Get Notifier Status(notifier=w1016) -> (notifier out=w1014:refnum<notifier>, current notification=w1011:T8)  [unwired: 1 in, 3 out]
            n79 = property class="Bool (strict)"(reference=w1015) -> ("Label.Text"=w1013:string)  [unwired: 1 in, 2 out]
            n80 = case shown="\"XY Correction Active\"" w1013 {
              tunnel: w1012 -> [_ w1020 w1023 w1026]
              tunnel: w1011 -> [w1018 w1021 w1024 w1027]
              tunnel: [w1018 w1019 w1022 w1025] -> w1010
              frame Default {
              }
              frame "XY Correction Active" {
                n81 = Bundle By Name(cluster=w1021, "XY Correction Active"=w1020) -> (w1019:T8)
              }
              frame "Z Correction Active" {
                n82 = Bundle By Name(cluster=w1024, "Z Correction Active"=w1023) -> (w1022:T8)
              }
              frame "Abort If Error" {
                n83 = Bundle By Name(cluster=w1027, "Abort If Error"=w1026) -> (w1025:T8)
              }
            }
            n84 = Bundle By Name(cluster=w1010, "Actions"=4Pi_Obj_Lock_-_Actions."Idle") -> (w1008:T8)
            n85 = Send Notification(notification=w1008, notifier=w1014) -> ()  [unwired: 1 in, 2 out]
          }
          event "Z Drift Threshold", "Z Stage Move Limit (µm)", "XY Drift Threshold", "XY Stage Move Limit (µm)", "P (Proportional)", "I (Integral)", "D (Derivative)", "Sample Z Step Size (µm)": Value Change {
            n86 = event-data() -> ("NewVal"=w1032:dbl, "CtlRef"=w1033:refnum<vi>)  [unwired: 1 in]
            n87 = Get Notifier Status(notifier=w1034) -> (notifier out=w1031:refnum<notifier>, current notification=w1035:T8)  [unwired: 1 in, 3 out]
            n88 = property class="DigNum (strict)"(reference=w1033) -> ("Label.Text"=w1036:string)  [unwired: 1 in, 2 out]
            n89 = case shown="\"Sample Z Step Size (µm)\"" w1036 {
              tunnel: w1032 -> [_ w1040 w1043 w1046 w1049 w1054 w1060 w1066 w1070]
              tunnel: w1035 -> [w1038 w1041 w1044 w1047 w1050 w1053 w1059 w1065 w1071]
              tunnel: [w1038 w1039 w1042 w1045 w1048 w1051 w1057 w1063 w1069] -> w1029
              frame Default {
              }
              frame "Z Drift Threshold" {
                n90 = Bundle By Name(cluster=w1041, "Z Drift Threshold"=w1040) -> (w1039:T8)
              }
              frame "Z Stage Move Limit (µm)" {
                n91 = Bundle By Name(cluster=w1044, "Z Stage Move Limit (µm)"=w1043) -> (w1042:T8)
              }
              frame "XY Drift Threshold" {
                n92 = Bundle By Name(cluster=w1047, "XY Drift Threshold"=w1046) -> (w1045:T8)
              }
              frame "XY Stage Move Limit (µm)" {
                n93 = Bundle By Name(cluster=w1050, "XY Stage Move Limit (µm)"=w1049) -> (w1048:T8)
              }
              frame "P (Proportional)" {
                n94 = Unbundle By Name(w1053) -> ("PID Values"=w1056:dbl[])
                n95 = Replace Array Subset(array=w1056, new element=w1054, index=0) -> (w1052:dbl[])
                n96 = Bundle By Name(cluster=w1053, "PID Values"=w1052) -> (w1051:T8)
              }
              frame "I (Integral)" {
                n97 = Unbundle By Name(w1059) -> ("PID Values"=w1062:dbl[])
                n98 = Replace Array Subset(array=w1062, new element=w1060, index=1) -> (w1058:dbl[])
                n99 = Bundle By Name(cluster=w1059, "PID Values"=w1058) -> (w1057:T8)
              }
              frame "D (Derivative)" {
                n100 = Unbundle By Name(w1065) -> ("PID Values"=w1068:dbl[])
                n101 = Replace Array Subset(array=w1068, new element=w1066, index=2) -> (w1064:dbl[])
                n102 = Bundle By Name(cluster=w1065, "PID Values"=w1064) -> (w1063:T8)
              }
              frame "Sample Z Step Size (µm)" {
                n103 = Bundle By Name(cluster=w1071, "Z Step Size (µm)"=w1070) -> (w1069:T8)
              }
            }
            n104 = Bundle By Name(cluster=w1029, "Actions"=4Pi_Obj_Lock_-_Actions."Idle") -> (w1028:T8)
            n105 = Send Notification(notification=w1028, notifier=w1031) -> ()  [unwired: 1 in, 2 out]
          }
          event "Sample Z Step No.": Value Change {
            n106 = event-data() -> ("NewVal"=w1073:u32)  [unwired: 1 in]
            n107 = for {
              N: w1073 -> [_]
              tunnel: [w1092] -> w1077 mode=indexing
              tunnel: [w1081] -> w1076 mode=indexing
              i -> [w1091]
              w1082 = T12 3 items=["Grayscale (U8)", "Grayscale (I16)", "Grayscale (SGL)", "Complex (CSG)", "RGB (U32)", "HSL (U32)", "RGB (U64)", "Grayscale (U16)"] ("Image Type")
              w1087 = T12 2 items=["Grayscale (U8)", "Grayscale (I16)", "Grayscale (SGL)", "Complex (CSG)", "RGB (U32)", "HSL (U32)", "RGB (U64)", "Grayscale (U16)"] ("Image Type")
              w1083 = 10 ("Border Size")
              n108 = Number To Decimal String(number=w1091, width (-)=i16 1) -> (decimal integer string=w1089:string)
              n109 = Concatenate Strings("Ref Stack " ("string"), w1089) -> (w1085:string)
              n110 = call "IMAQ Create"("Border Size"=w1083, "Image Name"=w1085, "Image Type"=w1087) -> ("New Image"=w1092:T9)  [unwired: 2 in, 1 out]
              n111 = Concatenate Strings("FFT" ("string"), w1085) -> (w1084:string)
              n112 = call "IMAQ Create"("Border Size"=w1083, "Image Name"=w1084, "Image Type"=w1082) -> ("New Image"=w1081:T9)  [unwired: 2 in, 1 out]
            }
            n113 = Get Notifier Status(notifier=w1075) -> (notifier out=w1079:refnum<notifier>, current notification=w1080:T8)  [unwired: 1 in, 3 out]
            n114 = Bundle By Name(cluster=w1080, "Actions"=4Pi_Obj_Lock_-_Actions."Idle", "Z Step No."=w1073, "Ref Stack (SGL)"=w1077, "Ref FFT Stack (CSG)"=w1076) -> (w1078:T8)
            n115 = Send Notification(notification=w1078, notifier=w1079) -> ()  [unwired: 1 in, 2 out]
          }
          event "Frame Accumulations": Value Change {
            n116 = event-data() -> ("NewVal"=w1095:u16)  [unwired: 1 in]
            n117 = Get Notifier Status(notifier=w1098) -> (notifier out=w1097:refnum<notifier>, current notification=w1096:T8)  [unwired: 1 in, 3 out]
            n118 = Bundle By Name(cluster=w1096, "Actions"=4Pi_Obj_Lock_-_Actions."Idle", "Frame Accumulations"=w1095) -> (w1094:T8)
            n119 = Send Notification(notification=w1094, notifier=w1097) -> ()  [unwired: 1 in, 2 out]
          }
          event "Update Delay (ms)": Value Change {
            n120 = event-data() -> ("NewVal"=w1102:i32)  [unwired: 1 in]
            n121 = Get Notifier Status(notifier=w1105) -> (notifier out=w1104:refnum<notifier>, current notification=w1103:T8)  [unwired: 1 in, 3 out]
            n122 = Bundle By Name(cluster=w1103, "Actions"=4Pi_Obj_Lock_-_Actions."Idle", "Update Delay (ms)"=w1102) -> (w1101:T8)
            n123 = Send Notification(notification=w1101, notifier=w1104) -> ()  [unwired: 1 in, 2 out]
          }
          event "Save Lock Settings": Value Change {
            n124 = event-data() -> ()  [unwired: 1 in, 1 out]
            n125 = Wait on Notification(notifier=w1134) -> (notification=w1132:T8)  [unwired: 3 in, 3 out]
            n126 = Unbundle By Name(w1132) -> ("Z Step Size (µm)"=w1108:dbl, "Z Step No."=w1107:u32, "Z Drift Threshold"=w1131:dbl, "Z Stage Move Limit (µm)"=w1130:dbl, "XY Drift Threshold"=w1129:dbl, "XY Stage Move Limit (µm)"=w1128:dbl, "Frame Accumulations"=w1127:u16, "Abort If Error"=w1126:bool, "Z Correction Active"=w1125:bool, "XY Correction Active"=w1124:bool, "PID Values"=w1114:dbl[])
            n127 = local read "Invert X Axis"() -> (w1112:bool)
            n128 = local read "Invert Y Axis"() -> (w1111:bool)
            n129 = local read "Invert Z Axis"() -> (w1110:bool)
            n130 = local read "Flip XY Axis"() -> (w1113:bool)
            n131 = Bundle By Name(cluster=T7 {"Z Drift Threshold"=0.05, "Z Stage Move Limit (µm)"=1.0, "XY Drift Threshold"=0.05, "XY Stage Move Limit (µm)"=1.0, "Frame Accumulations"=10, "Abort If Error"=FALSE, "Flip XY Axis"=FALSE, "Invert X Axis"=FALSE, "Invert Y Axis"=FALSE, "Invert Z Axis"=FALSE, "Z Correction Active"=TRUE, "XY Correction Active"=TRUE, "PID Values"=[], "Update Delay (ms)"=0, "Sample Z Step Size (µm)"=2.0, "Sample Z Step No."=2, "Z Update Scale Factor"=2.0, "Y Update Scale Factor"=2.0, "X Update Scale Factor"=2.0} ("Lock Settings"), "Sample Z Step Size (µm)"=w1108, "Sample Z Step No."=w1107, "Z Drift Threshold"=w1131, "Z Stage Move Limit (µm)"=w1130, "XY Drift Threshold"=w1129, "XY Stage Move Limit (µm)"=w1128, "Frame Accumulations"=w1127, "Abort If Error"=w1126, "Z Correction Active"=w1125, "XY Correction Active"=w1124, "PID Values"=w1114, "Flip XY Axis"=w1113, "Invert X Axis"=w1112, "Invert Y Axis"=w1111, "Invert Z Axis"=w1110) -> (w1123:T7)
            n132 = control-ref of="This VI"() -> (w1121:refnum<vi>)
            n133 = Flatten To JSON(anything=w1123) -> (JSON string=w1116:string)  [unwired: 2 in, 1 out]
            n134 = property class="VI"(reference=w1121) -> ("Path"=w1118:path)  [unwired: 1 in, 2 out]
            n135 = Strip Path(path=w1118) -> (stripped path=w1117:path)  [unwired: 1 out]
            n136 = Build Path(base path=w1117, name or relative path="4Pi Objective Lock Default Settings") -> (appended path=w1119:path)
            n137 = Build Path(base path=w1119, name or relative path="Default Obj Lock Settings.json") -> (appended path=w1115:path)
            n138 = Write to Text File(file (use dialog)=w1115, text=w1116) -> (refnum out=w1109:refnum<file>)  [unwired: 2 in, 2 out]
            n139 = Close File(refnum=w1109) -> ()  [unwired: 1 in, 2 out]
          }
          event "Start Lock": Value Change {
            n140 = event-data() -> ("NewVal"=w1141:bool)  [unwired: 1 in]
            n141 = Select(t=4Pi_Obj_Lock_-_Actions."Start Lock", s=w1141, f=4Pi_Obj_Lock_-_Actions."Abort" ("Actions")) -> (s? t:f=w1139:T6)
            n142 = Get Notifier Status(notifier=w1144) -> (notifier out=w1143:refnum<notifier>, current notification=w1142:T8)  [unwired: 1 in, 3 out]
            n143 = Bundle By Name(cluster=w1142, "Actions"=w1139, "Running?"=TRUE) -> (w1138:T8)
            n144 = Send Notification(notification=w1138, notifier=w1143) -> ()  [unwired: 1 in, 2 out]
          }
          event "Restart Lock": Value Change {
            n145 = event-data() -> ()  [unwired: 1 in, 1 out]
            n146 = Get Notifier Status(notifier=w1151) -> (notifier out=w1150:refnum<notifier>, current notification=w1149:T8)  [unwired: 1 in, 3 out]
            n147 = Bundle By Name(cluster=w1149, "Actions"=4Pi_Obj_Lock_-_Actions."Restart Lock" ("t")) -> (w1148:T8)
            n148 = local write "Start Lock"(TRUE ("Start Lock")) -> ()
            n149 = Send Notification(notification=w1148, notifier=w1150) -> ()  [unwired: 1 in, 2 out]
          }
          event "Quit": Value Change {
            # "Turn off the OBJ lock before quiting."
            n150 = event-data() -> ("NewVal"=w1162:bool)  [unwired: 1 in]
            n151 = Get Notifier Status(notifier=w1157) -> (notifier out=w1155:refnum<notifier>, current notification=w1153:T8)  [unwired: 1 in, 3 out]
            n152 = Unbundle By Name(w1153) -> ("Running?"=w1156:bool)
            n153 = case shown="True" w1156 {
              tunnel: w1155 -> [w1163 w1167]
              tunnel: [w1163 w1164] -> w1154
              tunnel: w1153 -> [_ w1169]
              frame False {
              }
              frame True {
                n154 = Bundle By Name(cluster=w1169, "Actions"=4Pi_Obj_Lock_-_Actions."Abort") -> (w1166:T8)
                n155 = Send Notification(notification=w1166, notifier=w1167) -> (notifier out=w1165:refnum<notifier>)  [unwired: 1 in, 1 out]
                n156 = while {
                  tunnel: w1165 -> [w1179]
                  tunnel: [w1174] -> w1164
                  i -> [w1173]
                  stop <- w1175 stop-if-true
                  n157 = Get Notifier Status(notifier=w1179) -> (notifier out=w1174:refnum<notifier>, # waiting=w1178:i32)  [unwired: 1 in, 3 out]
                  n158 = Greater?(x=w1173, y=1500) -> (0:w1171:bool)
                  n159 = Less?(x=w1178, y=1) -> (x < y?=w1176:bool)
                  n160 = Or(x=w1176, y=w1171) -> (x .or. y?=w1175:bool)
                  n161 = Wait (ms)(milliseconds to wait=u32 1) -> ()  [unwired: 1 out]
                }
              }
            }
            n162 = Get Notifier Status(notifier=w1154) -> (notifier out=w1159:refnum<notifier>, current notification=w1161:T8)  [unwired: 1 in, 3 out]
            n163 = Bundle By Name(cluster=w1161, "Actions"=4Pi_Obj_Lock_-_Actions."Quit") -> (w1158:T8)
            n164 = Send Notification(notification=w1158, notifier=w1159) -> ()  [unwired: 1 in, 2 out]
          }
        }
      }
      n165 = while {
        tunnel: w196 -> [w222]
        tunnel: w194 -> [w210]
        tunnel: w193 -> [w209]
        tunnel: w195 -> [w221]
        stop <- w217 stop-if-true
        # "Column 1 - Target Lock Values\nColumn 2 - Current Values\nColumn 3 - Differnce Values\nColumn 4 - Initial XYZ Stage Positions"
        n166 = Wait on Notification(notifier=w221, ignore previous (F)=FALSE) -> (notifier out=w216:refnum<notifier>, notification=w219:T8)  [unwired: 2 in, 2 out]
        n167 = Unbundle By Name(w219) -> ("Actions"=w211:T6)
        n168 = Equal?(x=4Pi_Obj_Lock_-_Actions."Quit", y=w211) -> (x = y?=w217:bool)
        n169 = Initialize Array(0.0 ("element"), 3 ("dimension size"), 4 ("dimension size")) -> (w213:dbl[][])
        n170 = while {
          shift-right: [w229] -> _
          shift-left: w211 -> [w237]
          tunnel: w222 -> [w241]
          tunnel: w210 -> [w240]
          tunnel: w209 -> [w239]
          tunnel: w216 -> [w235]
          shift-right: [w223] -> _
          shift-left: w213 -> [w224]
          stop <- w236 stop-if-true
          w231 = 4Pi_Obj_Lock_-_Actions."Abort" ("x")
          n171 = case shown="\"Delay\"" w237 {
            selector: w237 -> [_ _ _ _ _ _ _ _ _ _ _ _ _ w776 _ _ _ _ _ _]
            tunnel: w241 -> [_ w251 _ w358 _ _ w468 w511 w554 _ w619 _ _ _ _ _ _ w961 _ _]
            tunnel: w240 -> [_ w285 _ _ _ _ w444 _ _ _ _ _ _ w780 _ _ _ _ _ _]
            tunnel: w239 -> [_ w284 w314 w359 _ w419 w443 _ _ _ _ _ _ _ w854 _ _ _ _ _]
            tunnel: FALSE -> [w244 w297 w310 w357 w397 w415 w471 w542 w556 w591 w649 w694 w706 w806 w859 w939 w948 w965 _ _]
            tunnel: [4Pi_Obj_Lock_-_Actions."Exit Loop" ("x") w247 4Pi_Obj_Lock_-_Actions."Get Ref Stack" ("x") w362 4Pi_Obj_Lock_-_Actions."Move To Init Z" ("x") 4Pi_Obj_Lock_-_Actions."Get Initial Position" ("x") w463 w525 w559 4Pi_Obj_Lock_-_Actions."Get Current Position" ("x") w636 w672 w710 w795 w835 4Pi_Obj_Lock_-_Actions."Delay" ("x") 4Pi_Obj_Lock_-_Actions."Get Current Z Position" ("x") 4Pi_Obj_Lock_-_Actions."Exit Loop" ("x") 4Pi_Obj_Lock_-_Actions."Exit Loop" ("x") 4Pi_Obj_Lock_-_Actions."Quit" ("x")] -> w230
            tunnel: [w244 w297 w310 w357 w397 w415 w471 w542 w556 w591 w649 w694 w706 w806 w859 w939 w948 w965 TRUE TRUE] -> w236
            tunnel: w235 -> [w243 w268 w315 w361 w402 w413 w470 w541 w566 w614 w648 w693 w741 w805 w857 w937 w946 w969 w975 w979]
            tunnel: [w243 w262 w313 w360 w399 w413 w470 w533 w565 w589 w647 w692 w709 w804 w856 w936 w942 w968 w975 w978] -> w234
            tunnel: w224 -> [w242 w281 w309 w356 w396 w414 w456 w540 w555 w590 w624 w682 w705 w766 w833 w917 w945 w964 w974 w987]
            tunnel: [w242 w280 w309 w356 w396 w414 w455 w539 w555 w590 w623 w679 w705 w766 w833 w917 w945 w964 w974 w987] -> w223
            frame "Idle", Default {
            }
            frame "Start Lock" {
              w261 = T17 [] ("History Data")
              w277 = FALSE ("Move Limit Error")
              w282 = Stage_Actions."Get Position" ("Actions")
              n172 = control-ref of="This VI"() -> (w295:refnum<vi>)
              n173 = call "Stages Messenger.vi"("Stage Notifier Name"=w285, "Actions"=w282) -> ("Positions"=w286:dbl[])  [unwired: 10 in, 3 out]
              n174 = call "Stages Messenger.vi"("Stage Notifier Name"=w284, "Actions"=w282) -> ("Positions"=w287:dbl[])  [unwired: 10 in, 3 out]
              n175 = property class="VI"(reference=w295) -> ("Path"=w292:path)  [unwired: 1 in, 2 out]
              n176 = local write "Move Limit Error"(w277) -> ()
              n177 = local write "Fit Error"(w277) -> ()
              n178 = Index Array(array=w287, index=0) -> (element=w283:dbl)
              n179 = Strip Path(path=w292) -> (stripped path=w291:path)  [unwired: 1 out]
              n180 = Build Path(base path=w291, name or relative path="4Pi Objective Lock Default Settings") -> (appended path=w293:path)
              n181 = Build Array (concatenate)(w286, w283) -> (w260:dbl[])
              n182 = Build Path(base path=w293, name or relative path="Initial Stage Positions.json") -> (appended path=w289:path)
              n183 = Flatten To JSON(anything=w260) -> (JSON string=w290:string)  [unwired: 2 in, 1 out]
              n184 = Replace Array Subset(array=w281, new element=w260, index (col)=3 ("disabled index (col)")) -> (w280:dbl[][])  [unwired: 1 in]
              n185 = Index Array(array=w260, index #1=0 ("index"), index #2=1 ("index"), index #3=2 ("index")) -> (element #1=w256:dbl, element #2=w254:dbl, element #3=w255:dbl)
              n186 = Write to Text File(file (use dialog)=w289, text=w290) -> (refnum out=w278:refnum<file>)  [unwired: 2 in, 2 out]
              n187 = local write "X Axis Position (µm)"(w256) -> ()
              n188 = local write "Y Axis Position (µm)"(w254) -> ()
              n189 = local write "Z Axis Position (µm)"(w255) -> ()
              n190 = Get Notifier Status(notifier=w268) -> (notifier out=w262:refnum<notifier>, current notification=w267:T8)  [unwired: 1 in, 3 out]
              n191 = Close File(refnum=w278) -> ()  [unwired: 1 in, 2 out]
              n192 = Unbundle By Name(w267) -> ("Cur Image (SGL)"=w266:T9)
              n193 = Unbundle By Name(w267) -> ("Z Step No."=w264:u32, "Ref Stack (SGL)"=w263:T9[])
              n194 = call "Camera Messenger.vi"("Notifier Name"=w251, "General Camera Actions"=Generic_Camera_Actions."Live Preview") -> ("Notifier Name Dup"=w252:string)  [unwired: 8 in, 5 out]
              n195 = while {
                tunnel: w252 -> [w305]
                tunnel: [w300] -> w249
                tunnel: [w298] -> w250
                i -> [w304]
                stop <- w301 stop-if-true
                n196 = call "Camera Messenger.vi"("Notifier Name"=w305, "General Camera Actions"=Generic_Camera_Actions."Status") -> ("Notifier Name Dup"=w298:string, "Running?"=w302:bool)  [unwired: 8 in, 4 out]
                n197 = Greater?(x=w304, y=3000) -> (0:w300:bool)
                n198 = Or(x=w302, y=w300) -> (x .or. y?=w301:bool)
                n199 = Wait (ms)(milliseconds to wait=u32 1) -> ()  [unwired: 1 out]
              }
              n200 = call "Camera Messenger.vi"("Notifier Name"=w250, "General Camera Actions"=Generic_Camera_Actions."Get ROI", "Camera ROI"=T14 {"H_Offset"=0, "V_Offset"=0, "H_Width"=0, "V_Width"=0} ("General Camera ROI")) -> ("Camera ROI"=w269:T14)  [unwired: 7 in, 5 out]
              n201 = Unbundle By Name(w269) -> ("H_Width"=w274:u16, "V_Width"=w272:u16)
              n202 = To Long Integer(number=w274) -> (32bit integer=w273:i32)
              n203 = To Long Integer(number=w272) -> (32bit integer=w271:i32)
              n204 = Initialize Array(sgl 0.0 ("element"), w273, w271) -> (w265:sgl[][])
              n205 = for {
                N: w264 -> [_]
                tunnel: w265 -> [w307]
                tunnel: w263 -> [w308] mode=indexing
                n206 = call "IMAQ ArrayToImage"("Image Pixels (Float)"=w307, "Image"=w308) -> ()  [unwired: 8 in, 2 out]
              }
              n207 = call "IMAQ ArrayToImage"("Image Pixels (Float)"=w265, "Image"=w266) -> ()  [unwired: 8 in, 2 out]
              n208 = property on="X Target and Fit Position (µm)" class="WFChart (strict)"("History Data"=w261) -> ()  [unwired: 2 in, 2 out]
              n209 = property on="Y Target and Fit Position (µm)" class="WFChart (strict)"("History Data"=w261) -> ()  [unwired: 2 in, 2 out]
              n210 = property on="Z Target and Fit Value (µm)" class="WFChart (strict)"("History Data"=w261) -> ()  [unwired: 2 in, 2 out]
              n211 = Select(t=4Pi_Obj_Lock_-_Actions."Exit Loop", s=w249, f=4Pi_Obj_Lock_-_Actions."Get Target Z Position" ("x")) -> (s? t:f=w247:T6)
            }
            frame "Get Target Z Position" {
              w337 = 0.0 ("Target Z (µm)")
              n212 = Get Notifier Status(notifier=w315) -> (notifier out=w335:refnum<notifier>, current notification=w340:T8)  [unwired: 1 in, 3 out]
              n213 = Unbundle By Name(w340) -> ("Z Step No."=w333:u32, "Z Step Size (µm)"=w332:dbl, "Z Stage Move Limit (µm)"=w330:dbl)
              n214 = Unbundle By Name(w340) -> ("Z Step No."=w325:u32, "Z Step Size (µm)"=w338:dbl)
              n215 = Divide(x=w333, y=2.0) -> (x/y=w323:dbl)
              n216 = Round Toward -Infinity(1:w323) -> (0:w322:dbl)
              n217 = Multiply(x=w322, y=w332) -> (x*y=w327:dbl)
              n218 = Decrement(x=w325) -> (x-1=w324:u32)
              n219 = Negate(x=w327) -> (-x=w326:dbl)
              n220 = Negate(x=w330) -> (-x=w331:dbl)
              n221 = In Range and Coerce(upper limit=w330, x=w326, lower limit=w331) -> (coerced(x)=w328:dbl)  [unwired: 1 out]
              n222 = Add(x=w337, y=w328) -> (x+y=w329:dbl)
              n223 = Build Array(w329) -> (w339:dbl[])
              n224 = for {
                N: w324 -> [_]
                tunnel: w338 -> [w351]
                shift-right: [w352] -> w336
                shift-left: w339 -> [w353]
                shift-right: [w349] -> _
                shift-left: w329 -> [w350]
                n225 = Add(x=w350, y=w351) -> (x+y=w349:dbl)
                n226 = Build Array (concatenate)(w353, w349) -> (w352:dbl[])
              }
              n227 = Build Array(w328) -> (w341:dbl[])
              n228 = call "Stages Messenger.vi"("Stage Notifier Name"=w314, "Actions"=Stage_Actions."MVR", "Setpoint"=w341, "Axis"=bool[] [TRUE], "Exit While Busy?"=TRUE) -> ("Stage Notifier Name (Dup)"=w320:string, "Status"=w321:T18)  [unwired: 7 in, 2 out]
              n229 = case shown="Default" w321 {
                tunnel: [w347] -> w319
                tunnel: w320 -> [w347]
                frame Default {
                  n230 = Wait (ms)(milliseconds to wait=u32 250) -> ()  [unwired: 1 out]
                }
              }
              n231 = Bundle By Name(cluster=w340, "Sample Z (µm)"=w336) -> (w334:T8)
              n232 = call "Stages Messenger.vi"("Stage Notifier Name"=w319, "Actions"=Stage_Actions."Get Position", "Exit While Busy?"=TRUE) -> ("Positions"=w317:dbl[])  [unwired: 9 in, 3 out]
              n233 = Index Array(array=w317, index=0) -> (element=w311:dbl)
              n234 = Send Notification(notification=w334, notifier=w335) -> (notifier out=w313:refnum<notifier>)  [unwired: 1 in, 1 out]
              n235 = local write "Z Axis Position (µm)"(w311) -> ()
              "Target Z (µm)" <- w337
            }
            frame "Get Ref Stack" {
              n236 = Get Notifier Status(notifier=w361) -> (notifier out=w360:refnum<notifier>, current notification=w355:T8)  [unwired: 1 in, 3 out]
              n237 = Unbundle By Name(w355) -> ("Z Step No."=w365:u32, "Ref Stack (SGL)"=w364:T9[])
              n238 = Unbundle By Name(w355) -> ("Frame Accumulations"=w354:u16)
              n239 = Unbundle By Name(w355) -> ("Z Step Size (µm)"=w363:dbl)
              n240 = while {
                tunnel: w358 -> [w383]
                tunnel: w365 -> [w380]
                tunnel: w360 -> [w382]
                tunnel: [w372] -> w362
                tunnel: w364 -> [w371] mode=indexing
                tunnel: w363 -> [w370]
                tunnel: w359 -> [w369]
                tunnel: w354 -> [w366]
                i -> [w379]
                stop <- w375 stop-if-true
                n241 = flat-sequence {
                  tunnel: w383 -> [w386]
                  tunnel: w371 -> [w384]
                  tunnel: w366 -> [w385]
                  tunnel: w370 -> [w390]
                  tunnel: w369 -> [w389]
                  frame #0 {
                    n242 = call "Generic Camera Get New Camera Image.vi"("Camera Notifier Name"=w386, "Frames"=w385) -> ("Image - U16"=w388:u16[][])  [unwired: 11 in, 2 out]
                    n243 = To Single Precision Float(number=w388) -> (single precision float=w387:sgl[][])
                    n244 = call "IMAQ ArrayToImage"("Image Pixels (Float)"=w387, "Image"=w384) -> ()  [unwired: 8 in, 2 out]
                  }
                  frame #1 {
                    n245 = Build Array(w390) -> (w394:dbl[])
                    n246 = Wait (ms)(milliseconds to wait=u32 250) -> ()  [unwired: 1 out]
                    n247 = call "Stages Messenger.vi"("Stage Notifier Name"=w389, "Actions"=Stage_Actions."MVR", "Setpoint"=w394, "Axis"=bool[] [TRUE], "Exit While Busy?"=TRUE) -> ()  [unwired: 7 in, 4 out]
                  }
                }
                n248 = Get Notifier Status(notifier=w382) -> (current notification=w374:T8)  [unwired: 1 in, 4 out]
                n249 = To Unsigned Long Integer(number=w379) -> (unsigned 32bit integer=w378:u32)
                n250 = Increment(x=w378) -> (x+1=w381:u32)
                n251 = Unbundle By Name(w374) -> ("Running?"=w377:bool)
                n252 = Greater Or Equal?(x=w381, y=w380) -> (x >= y?=w376:bool)
                n253 = Not(x=w377) -> (.not. x?=w373:bool)
                n254 = Or(x=w373, y=w376) -> (x .or. y?=w375:bool)
                n255 = Select(t=4Pi_Obj_Lock_-_Actions."Abort" ("x"), s=w373, f=4Pi_Obj_Lock_-_Actions."Cal Ref FFT") -> (s? t:f=w372:T6)
              }
            }
            frame "Cal Ref FFT" {
              n256 = Get Notifier Status(notifier=w402) -> (notifier out=w399:refnum<notifier>, current notification=w403:T8)  [unwired: 1 in, 3 out]
              n257 = Unbundle By Name(w403) -> ("Ref Stack (SGL)"=w401:T9[], "Ref FFT Stack (CSG)"=w400:T9[])
              n258 = for {
                tunnel: w401 -> [w405] mode=indexing
                tunnel: w400 -> [w404] mode=indexing
                n259 = call "4Pi Obj Lock - Norm FFT.vi"("FFT Image Dst"=w404, "Image In"=w405) -> ()  [unwired: 8 in, 2 out]
              }
            }
            frame "Move To Init Z" {
              # "initial z stage position"
              n260 = Index Array(array=w414, index (row)=2, index (col)=3 ("disabled index (col)")) -> (element=w416:dbl)
              n261 = flat-sequence {
                tunnel: w419 -> [w429]
                tunnel: [w428] -> w421
                tunnel: w416 -> [w424]
                tunnel: [w422] -> w420
                tunnel: w421 -> [w434]
                tunnel: w420 -> [w433]
                tunnel: [w432] -> w407
                frame #0 {
                  n262 = call "Stages Messenger.vi"("Stage Notifier Name"=w429, "Actions"=Stage_Actions."Get Position") -> ("Stage Notifier Name (Dup)"=w428:string, "Positions"=w426:dbl[])  [unwired: 10 in, 2 out]
                  n263 = Index Array(array=w426, index=0) -> (element=w425:dbl)
                  n264 = Subtract(x=w424, y=w425) -> (x-y=w423:dbl)
                  n265 = Build Array(w423) -> (w422:dbl[])
                }
                frame #1 {
                  n266 = Wait (ms)(milliseconds to wait=u32 250) -> ()  [unwired: 1 out]
                  n267 = call "Stages Messenger.vi"("Stage Notifier Name"=w434, "Actions"=Stage_Actions."MVR", "Setpoint"=w433, "Axis"=bool[] [TRUE], "Exit While Busy?"=TRUE) -> ("Stage Notifier Name (Dup)"=w432:string)  [unwired: 7 in, 3 out]
                }
              }
              n268 = call "Stages Messenger.vi"("Stage Notifier Name"=w407, "Actions"=Stage_Actions."Get Position", "Exit While Busy?"=TRUE) -> ("Positions"=w410:dbl[])  [unwired: 9 in, 3 out]
              n269 = Index Array(array=w410, index=0) -> (element=w408:dbl)
              n270 = local write "Z Axis Position (µm)"(w408) -> ()
            }
            frame "Restart Lock" {
              w438 = T17 [] ("History Data")
              w439 = FALSE ("Move Limit Error")
              # "Make sure the camera is running, if not abort."
              n271 = control-ref of="This VI"() -> (w461:refnum<vi>)
              n272 = call "Camera Messenger.vi"("Notifier Name"=w468, "General Camera Actions"=Generic_Camera_Actions."Live Preview") -> ("Notifier Name Dup"=w467:string)  [unwired: 8 in, 5 out]
              n273 = property class="VI"(reference=w461) -> (error out=w447:errorcluster, "Path"=w458:path)  [unwired: 1 in, 1 out]
              n274 = while {
                tunnel: w467 -> [w497]
                tunnel: [w492] -> w466
                i -> [w496]
                stop <- w493 stop-if-true
                n275 = call "Camera Messenger.vi"("Notifier Name"=w497, "General Camera Actions"=Generic_Camera_Actions."Status") -> ("Running?"=w494:bool)  [unwired: 8 in, 5 out]
                n276 = Greater?(x=w496, y=3000) -> (0:w492:bool)
                n277 = Or(x=w494, y=w492) -> (x .or. y?=w493:bool)
                n278 = Wait (ms)(milliseconds to wait=u32 1) -> ()  [unwired: 1 out]
              }
              n279 = Strip Path(path=w458) -> (stripped path=w457:path)  [unwired: 1 out]
              n280 = Build Path(base path=w457, name or relative path="4Pi Objective Lock Default Settings") -> (appended path=w459:path)
              n281 = Build Path(base path=w459, name or relative path="Initial Stage Positions.json") -> (appended path=w453:path)
              n282 = Read from Text File(file (use dialog)=w453, error in=w447) -> (refnum out=w452:refnum<file>, text=w451:string, error out=w450:errorcluster)  [unwired: 2 in, 1 out]
              n283 = Close File(refnum=w452, error in=w450) -> (error out=w449:errorcluster)  [unwired: 1 out]
              n284 = local write "Move Limit Error"(w439) -> ()
              n285 = local write "Fit Error"(w439) -> ()
              n286 = Unflatten From JSON(JSON string=w451, type and defaults=dbl[] [], error in (no error)=w449) -> (value=w445:dbl[], error out=w446:errorcluster)  [unwired: 4 in]
              n287 = case shown="Error" w446 {
                tunnel: w445 -> [w473 _]
                tunnel: w444 -> [w480 w485]
                tunnel: w443 -> [w479 w484]
                tunnel: [w473 w483] -> w442
                tunnel: u32 150 ("milliseconds to wait") -> [w472 w482]
                tunnel: [w472 w482] -> w440
                frame No Error {
                  w481 = Stage_Actions."MOVE" ("Actions")
                  n288 = Split 1D Array(array=w473, index=2) -> (first subarray=w477:dbl[], second subarray=w476:dbl[])
                  n289 = call "Stages Messenger.vi"("Stage Notifier Name"=w480, "Actions"=w481, "Setpoint"=w477, "Axis"=bool[] [TRUE, TRUE]) -> ()  [unwired: 8 in, 4 out]
                  n290 = call "Stages Messenger.vi"("Stage Notifier Name"=w479, "Actions"=w481, "Setpoint"=w476, "Axis"=bool[] [TRUE]) -> ()  [unwired: 8 in, 4 out]
                }
                frame Error {
                  w486 = Stage_Actions."Get Position" ("Actions")
                  n291 = call "Stages Messenger.vi"("Stage Notifier Name"=w485, "Actions"=w486) -> ("Positions"=w488:dbl[])  [unwired: 10 in, 3 out]
                  n292 = call "Stages Messenger.vi"("Stage Notifier Name"=w484, "Actions"=w486) -> ("Positions"=w489:dbl[])  [unwired: 10 in, 3 out]
                  n293 = Index Array(array=w489, index=0) -> (element=w487:dbl)
                  n294 = Build Array (concatenate)(w488, w487) -> (w483:dbl[])
                }
              }
              n295 = Wait (ms)(milliseconds to wait=w440) -> ()  [unwired: 1 out]
              n296 = property on="X Target and Fit Position (µm)" class="WFChart (strict)"("History Data"=w438) -> ()  [unwired: 2 in, 2 out]
              n297 = property on="Y Target and Fit Position (µm)" class="WFChart (strict)"("History Data"=w438) -> ()  [unwired: 2 in, 2 out]
              n298 = property on="Z Target and Fit Value (µm)" class="WFChart (strict)"("History Data"=w438) -> ()  [unwired: 2 in, 2 out]
              n299 = Replace Array Subset(array=w456, new element=w442, index (col)=3 ("disabled index (col)")) -> (w455:dbl[][])  [unwired: 1 in]
              n300 = Select(t=4Pi_Obj_Lock_-_Actions."Exit Loop" ("x"), s=w466, f=4Pi_Obj_Lock_-_Actions."Get Initial Position" ("x")) -> (s? t:f=w463:T6)
            }
            frame "Get Initial Position" {
              w518 = 0 ("index")
              # "Set target values"
              n301 = Get Notifier Status(notifier=w541) -> (notifier out=w534:refnum<notifier>, current notification=w510:T8)  [unwired: 1 in, 3 out]
              n302 = Unbundle By Name(w510) -> ("Frame Accumulations"=w509:u16)
              n303 = Bundle By Name(cluster=w510, "Running?"=TRUE) -> (w531:T8)
              n304 = Send Notification(notification=w531, notifier=w534) -> (notifier out=w533:refnum<notifier>)  [unwired: 1 in, 1 out]
              n305 = call "Generic Camera Get New Camera Image.vi"("Camera Notifier Name"=w511, "Frames"=w509) -> ("Image - U16"=w504:u16[][])  [unwired: 11 in, 2 out]
              n306 = Array Size(array=w504) -> (size(s)=w505:i32[])
              n307 = To Double Precision Float(number=w505) -> (double precision float=w508:dbl[])
              n308 = call "2D Gaussian - Fit Image U16.vi"("Image In (U16)"=w504) -> ("Best Fit Params"=w538:T19, "Error Out"=w524:errorcluster)  [unwired: 13 in]
              n309 = Divide(x=w508, y=2.0 ("index")) -> (x/y=w506:dbl[])
              n310 = Unbundle By Name(w524) -> ("status"=w523:bool)
              n311 = Round Toward -Infinity(1:w506) -> (0:w503:dbl[])
              n312 = Cluster To Array(cluster=w538) -> (array=w537:dbl[])
              n313 = local write "Fit Error"(w523) -> ()
              n314 = Index Array(array=w503, index #1=0 ("index"), index #2=1 ("index")) -> (element #1=→"Target Y Position cc (px)":dbl, element #2=→"Target X Position cc (px)":dbl)
              n315 = Array Subset(array=w537, index=1, length=4) -> (w530:dbl[])
              n316 = Index Array(array=w530, index #1=0 ("index"), index #2=1 ("index"), index #3=2 ("index"), index #4=3 ("index")) -> (element #1=w512:dbl, element #2=w513:dbl, element #3=w520:dbl, element #4=w519:dbl)
              "Target X Position (px)" <- w512
              "Target Y Position (px)" <- w513
              n317 = Divide(x=w520, y=w519) -> (x/y=w514:dbl)
              "Target sx/sy" <- w514
              n318 = Replace Array Subset(array=w540, new element #1=w512, index (row) #1=0 ("disabled index (row)"), index (col) #1=w518, new element #2=w513, index (row) #2=1 ("disabled index (row)"), index (col) #2=w518, new element #3=w514, index (row) #3=2 ("disabled index (row)"), index (col) #3=w518) -> (w539:dbl[][])
              n319 = Select(t=4Pi_Obj_Lock_-_Actions."Abort" ("x"), s=w523, f=4Pi_Obj_Lock_-_Actions."Get Current Z Position" ("x")) -> (s? t:f=w525:T6)
            }
            frame "Get Current Z Position" {
              n320 = Get Notifier Status(notifier=w566) -> (notifier out=w565:refnum<notifier>, current notification=w553:T8)  [unwired: 1 in, 3 out]
              n321 = Unbundle By Name(w553) -> ("CC Image (SGL)"=w544:T9, "CC Image Max (SGL)"=w543:T9)
              n322 = Unbundle By Name(w553) -> ("Ref FFT Stack (CSG)"=w572:T9[])
              n323 = Unbundle By Name(w553) -> ("Cur Image (SGL)"=w549:T9, "Tmp Image FFT (CSG)"=w562:T9[])
              n324 = Unbundle By Name(w553) -> ("Sample Z (µm)"=w574:dbl[])
              n325 = Unbundle By Name(w553) -> ("Frame Accumulations"=w552:u16)
              n326 = call "Generic Camera Get New Camera Image.vi"("Camera Notifier Name"=w554, "Frames"=w552) -> ("Image - U16"=w551:u16[][])  [unwired: 11 in, 2 out]
              n327 = Index Array(array=w562, index #1=0 ("index"), index #2=1 ("index"), index #3=2 ("index")) -> (element #1=w560:T9, element #2=w546:T9, element #3=w545:T9)
              n328 = To Single Precision Float(number=w551) -> (single precision float=w548:sgl[][])
              n329 = call "IMAQ ArrayToImage"("Image Pixels (Float)"=w548, "Image"=w549) -> ("Image Out"=w550:T9)  [unwired: 8 in, 1 out]
              n330 = call "4Pi Obj Lock - Norm FFT.vi"("FFT Image Dst"=w560, "Image In"=w550) -> ("FFT Image Out"=w570:T9)  [unwired: 8 in, 1 out]
              n331 = call "IMAQ ComplexConjugate"("Image Src"=w570) -> ("Image Dst Out"=w569:T9)  [unwired: 3 in, 1 out]
              n332 = for {
                tunnel: [w579] -> w575 mode=indexing
                tunnel: w569 -> [w585]
                tunnel: w572 -> [w584] mode=indexing
                shift-right: [w579] -> _
                shift-left: sgl 0.0 ("Max CC") -> [w580]
                tunnel: w546 -> [w583]
                tunnel: w545 -> [w582]
                tunnel: w544 -> [w578]
                tunnel: w543 -> [w576]
                n333 = call "4Pi Obj Lock - Get Cross Correlation.vi"("Ref FFT image"=w584, "Cur FFT Image"=w585, "FFT CC image"=w583, "iFFT image"=w582, "CC image"=w578) -> ("Max CC"=w579:sgl, "CC image Out"=w577:T9)  [unwired: 8 in, 1 out]
                n334 = Greater?(x=w579, y=w580) -> (0:w581:bool)
                n335 = case shown="True" w581 {
                  tunnel: w577 -> [_ w587]
                  tunnel: w576 -> [_ w586]
                  frame False {
                  }
                  frame True {
                    n336 = call "IMAQ Copy"("Image Dst"=w586, "Image Src"=w587) -> ()  [unwired: 4 in, 2 out]
                  }
                }
              }
              n337 = To Double Precision Float(number=w575) -> (double precision float=w571:dbl[])
              n338 = call "4Pi Obj Lock - Find Peak Position.vi"("Fit Size"=2, "y"=w571, "x"=w574) -> ("Coerced Peak Position"=w568:dbl)  [unwired: 7 in, 1 out]
              "Measured Z (µm)" <- w568
              n339 = Not A Number/Path/Refnum?(number/path/refnum=w568) -> (NaN/Path/Refnum?=w567:bool)
              n340 = Select(t=4Pi_Obj_Lock_-_Actions."Get Current Z Position" ("x"), s=w567, f=4Pi_Obj_Lock_-_Actions."Get Current XY Position") -> (s? t:f=w559:T6)
            }
            frame "Get Current XY Position" {
              w601 = 3 ("edge size")
              n341 = Get Notifier Status(notifier=w614) -> (notifier out=w589:refnum<notifier>, current notification=w613:T8)  [unwired: 1 in, 3 out]
              n342 = Unbundle By Name(w613) -> ("CC Image Max (SGL)"=w612:T9)
              n343 = call "IMAQ ImageToArray"("Image"=w612) -> ("Image Pixels (Float)"=w598:sgl[][])  [unwired: 3 in, 4 out]
              n344 = call "4Pi Obj Lock - FFT shift 2D.vi"("Input image"=w598) -> ("fft shifted image"=w597:sgl[][])  [unwired: 10 in]
              n345 = call "4Pi Obj Lock - Crop Imag at Max.vi"("edge size"=w601, "Input array"=w597) -> ("Y"=w607:i32, "X"=w608:i32, "subarray"=w611:sgl[][])  [unwired: 6 in, 1 out]
              n346 = To Double Precision Float(number=w611) -> (double precision float=w610:dbl[][])
              n347 = Build Array(w608, w607) -> (w606:i32[])
              n348 = call "2D Gaussian - Fit Image DBL.vi"("Image In (DBL)"=w610) -> ("Best Fit Params"=w609:T19)  [unwired: 13 in, 1 out]
              n349 = To Double Precision Float(number=w606) -> (double precision float=w603:dbl[])
              n350 = Unbundle By Name(w609) -> ("X Position"=w605:dbl, "Y Position"=w604:dbl)
              n351 = Build Array(w605, w604) -> (w602:dbl[])
              n352 = To Double Precision Float(number=w601) -> (double precision float=w600:dbl)
              n353 = Subtract(x=w602, y=w600) -> (x-y=w599:dbl[])
              n354 = Add(x=w599, y=w603) -> (x+y=w594:dbl[])
              n355 = Index Array(array=w594, index #1=0 ("index"), index #2=1 ("index")) -> (element #1=→"Measured X Position cc (px)":dbl, element #2=→"Measured Y Position cc (px)":dbl)
            }
            frame "Get Current Position" {
              w628 = 1 ("index")
              # "retake current image"
              # "Update current values"
              n356 = Get Notifier Status(notifier=w648) -> (notifier out=w647:refnum<notifier>, current notification=w616:T8)  [unwired: 1 in, 3 out]
              n357 = Unbundle By Name(w616) -> ("Abort If Error"=w641:bool, "Cur Image (SGL)"=w618:T9)
              n358 = case shown="False" FALSE {
                tunnel: w619 -> [_ w658]
                tunnel: w618 -> [w652 w655]
                tunnel: w616 -> [_ w657]
                tunnel: [w650 w654] -> w615
                frame False {
                  n359 = call "IMAQ ImageToArray"("Image"=w652) -> ("Image Pixels (Float)"=w651:sgl[][])  [unwired: 3 in, 4 out]
                  n360 = To Unsigned Word Integer(number=w651) -> (unsigned 16bit integer=w650:u16[][])
                }
                frame True {
                  n361 = Unbundle By Name(w657) -> ("Frame Accumulations"=w656:u16)
                  n362 = call "Generic Camera Get New Camera Image.vi"("Camera Notifier Name"=w658, "Frames"=w656) -> ("Image - U16"=w654:u16[][])  [unwired: 11 in, 2 out]
                  n363 = To Single Precision Float(number=w654) -> (single precision float=w653:sgl[][])
                  n364 = call "IMAQ ArrayToImage"("Image Pixels (Float)"=w653, "Image"=w655) -> ()  [unwired: 8 in, 2 out]
                }
              }
              n365 = call "2D Gaussian - Fit Image U16.vi"("Image In (U16)"=w615) -> ("Best Fit Params"=w646:T19, "Error Out"=w642:errorcluster)  [unwired: 13 in]
              n366 = Unbundle By Name(w642) -> ("status"=w640:bool)
              "Fit Error" <- w640
              n367 = And(x=w641, y=w640) -> (x .and. y?=w639:bool)
              n368 = Cluster To Array(cluster=w646) -> (array=w645:dbl[])
              n369 = Array Subset(array=w645, index=1, length=4) -> (w629:dbl[])
              n370 = Index Array(array=w629, index #1=0 ("index"), index #2=1 ("index"), index #3=2 ("index"), index #4=3 ("index")) -> (element #1=w620:dbl, element #2=w621:dbl, element #3=w631:dbl, element #4=w630:dbl)
              "Measured X Position (px)" <- w620
              "Measured Y Position (px)" <- w621
              n371 = Divide(x=w631, y=w630) -> (x/y=w622:dbl)
              "Measured sx/sy" <- w622
              n372 = Select(t=4Pi_Obj_Lock_-_Actions."Abort" ("x"), s=w639, f=4Pi_Obj_Lock_-_Actions."Check Drift cc" ("x")) -> (s? t:f=w636:T6)
              n373 = Replace Array Subset(array=w624, new element #1=w620, index (row) #1=0 ("disabled index (row)"), index (col) #1=w628, new element #2=w621, index (row) #2=1 ("disabled index (row)"), index (col) #2=w628, new element #3=w622, index (row) #3=2 ("disabled index (row)"), index (col) #3=w628) -> (w623:dbl[][])
            }
            frame "Check Drift" {
              # "Update the PID difference between target values and current values"
              # "Check if Sigma X / Sigma Y is over the limit"
              # "Check if XY values are over the limit"
              n374 = Get Notifier Status(notifier=w693) -> (notifier out=w692:refnum<notifier>, current notification=w691:T8)  [unwired: 1 in, 3 out]
              n375 = Unbundle By Name(w691) -> ("Z Correction Active"=w668:bool, "XY Correction Active"=w670:bool, "XY Drift Threshold"=w661:dbl, "Z Drift Threshold"=w663:dbl, "PID Values"=w690:dbl[])
              n376 = Index Array(array=w682, index (col) #1=0 ("disabled index (col)"), index (col) #2=1 ("index (col)")) -> (element #1=w684:dbl[], element #2=w683:dbl[])  [unwired: 2 in]
              n377 = Array To Cluster(array=w690) -> (cluster=w664:T20)
              n378 = local read "pixel size (µm)"() -> (w660:dbl)
              n379 = Build Array(w664) -> (w689:T21)
              n380 = Divide(x=w661, y=w660) -> (x/y=w662:dbl)
              n381 = call-poly <vilib>:"PID.vi"("PID gains"=w689, "process variable"=w683, "setpoint"=w684) -> ("output"=w680:dbl[])  [unwired: 7 in, 1 out]
              n382 = Build Array(w662, w662, w663) -> (w687:dbl[])
              n383 = Replace Array Subset(array=w682, new element=w680, index (col)=2 ("disabled index (col)")) -> (w679:dbl[][])  [unwired: 1 in]
              n384 = Absolute Value(x=w680) -> (abs(x)=w688:dbl[])
              n385 = Greater?(x=w688, y=w687) -> (0:w678:bool[])
              n386 = Split 1D Array(array=w678, index=2) -> (first subarray=w676:bool[], second subarray=w675:bool[])
              n387 = Or Array Elements(Boolean array=w676) -> (logical OR=w671:bool)
              n388 = Or Array Elements(Boolean array=w675) -> (logical OR=w659:bool)
              n389 = And(x=w670, y=w671) -> (x .and. y?=w669:bool)
              n390 = And(x=w668, y=w659) -> (x .and. y?=w667:bool)
              n391 = Build Array(w669, w667) -> (w674:bool[])
              n392 = Boolean Array To Number(Boolean array=w674) -> (number=w673:u32)
              n393 = case shown="0, Default" w673 {
                tunnel: [4Pi_Obj_Lock_-_Actions."Update Plots" ("x") 4Pi_Obj_Lock_-_Actions."Move XY" ("x") 4Pi_Obj_Lock_-_Actions."Move Z" ("x") 4Pi_Obj_Lock_-_Actions."Move XYZ" ("x")] -> w672
                tunnel: [w695 TRUE FALSE w703] -> w666
                tunnel: [w695 FALSE TRUE w703] -> w665
                frame 0, Default {
                  w695 = FALSE
                  # "XYZ within limits, no move"
                }
                frame 1 {
                  # "X or Y outside limit, move XY"
                }
                frame 2 {
                  # "Sigma X / Y outside limit, move Z"
                }
                frame 3 {
                  w703 = TRUE
                  # "XYZ outside limit, move all"
                }
              }
              "XY Move" <- w666
              "Z Move" <- w665
            }
            frame "Check Drift cc" {
              n394 = Get Notifier Status(notifier=w741) -> (notifier out=w709:refnum<notifier>, current notification=w727:T8)  [unwired: 1 in, 3 out]
              n395 = Unbundle By Name(w727) -> ("XY Correction Active"=w717:bool, "XY Drift Threshold"=w744:dbl, "PID Values"=w742:dbl[])
              n396 = local read "Measured Y Position cc (px)"() -> (w738:dbl)
              n397 = local read "Measured X Position cc (px)"() -> (w739:dbl)
              n398 = Unbundle By Name(w727) -> ("Z Correction Active"=w718:bool, "Z Drift Threshold"=w720:dbl, "PID Values"=w726:dbl[])
              n399 = local read "Target X Position cc (px)"() -> (w737:dbl)
              n400 = local read "Target Y Position cc (px)"() -> (w736:dbl)
              n401 = Array To Cluster(array=w742) -> (cluster=w743:T20)
              n402 = local read "pixel size (µm)"() -> (w745:dbl)
              n403 = Array To Cluster(array=w726) -> (cluster=w725:T20)
              n404 = Build Array(w743) -> (w740:T21)
              n405 = Build Array(w737, w736) -> (w734:dbl[])
              n406 = Build Array(w739, w738) -> (w735:dbl[])
              n407 = local read "Measured Z (µm)"() -> (w722:dbl)
              n408 = local read "Target Z (µm)"() -> (w723:dbl)
              n409 = Divide(x=w744, y=w745) -> (x/y=w732:dbl)
              n410 = Subtract(x=w735, y=w734) -> (x-y=w733:dbl[])
              n411 = call-poly <vilib>:"PID.vi"("PID gains"=w740, "process variable"=w735, "setpoint"=w734) -> ("output"=→"dxy (px)":dbl[])  [unwired: 7 in, 1 out]
              n412 = Build Array(w732, w732) -> (w731:dbl[])
              n413 = Absolute Value(x=w733) -> (abs(x)=w730:dbl[])
              n414 = Subtract(x=w722, y=w723) -> (x-y=w724:dbl)
              n415 = call-poly <vilib>:"PID.vi"("PID gains"=w725, "process variable"=w722, "setpoint"=w723) -> ("output"=→"dz (µm)":dbl)  [unwired: 7 in, 1 out]
              n416 = Greater?(x=w730, y=w731) -> (0:w729:bool[])
              n417 = Absolute Value(x=w724) -> (abs(x)=w721:dbl)
              n418 = Or Array Elements(Boolean array=w729) -> (logical OR=w728:bool)
              n419 = Greater?(x=w721, y=w720) -> (0:w719:bool)
              n420 = And(x=w717, y=w728) -> (x .and. y?=w712:bool)
              n421 = And(x=w718, y=w719) -> (x .and. y?=w711:bool)
              n422 = Build Array(w712, w711) -> (w713:bool[])
              n423 = Boolean Array To Number(Boolean array=w713) -> (number=w714:u32)
              n424 = case shown="1" w714 {
                tunnel: [4Pi_Obj_Lock_-_Actions."Update Plots" ("x") 4Pi_Obj_Lock_-_Actions."Move XY" ("x") 4Pi_Obj_Lock_-_Actions."Move Z" ("x") 4Pi_Obj_Lock_-_Actions."Move XYZ" ("x")] -> w710
                tunnel: [w746 TRUE FALSE w754] -> w708
                tunnel: [w746 FALSE TRUE w754] -> w707
                frame 0, Default {
                  w746 = FALSE
                  # "XYZ within limits, no move"
                }
                frame 1 {
                  # "X or Y outside limit, move XY"
                }
                frame 2 {
                  # "Sigma X / Y outside limit, move Z"
                }
                frame 3 {
                  w754 = TRUE
                  # "XYZ outside limit, move all"
                }
              }
              n425 = local write "XY Move"(w708) -> ()
              n426 = local write "Z Move"(w707) -> ()
            }
            frame "Move XYZ", "Move XY" {
              w788 = 2.0
              # "Initial XY stage positions"
              # "Check if move will go beyond ±2 µm of the original positions"
              n427 = case shown="False" FALSE {
                tunnel: w766 -> [_ w809]
                tunnel: [w807 w808] -> w761
                frame False {
                  n428 = local read "dxy (px)"() -> (w807:dbl[])
                }
                frame True {
                  # "Get XY Diff Values"
                  n429 = Array Subset(array=w809, index (row)=0 ("index"), length (row)=2 ("length"), index (col)=2 ("index")) -> (w810:dbl[][])  [unwired: 1 in]
                  n430 = Index Array(array=w810, index (col)=0 ("disabled index (col)")) -> (element=w808:dbl[])  [unwired: 1 in]
                }
              }
              n431 = Get Notifier Status(notifier=w805) -> (notifier out=w804:refnum<notifier>, current notification=w803:T8)  [unwired: 1 in, 3 out]
              n432 = Unbundle By Name(w803) -> ("Abort If Error"=w796:bool, "XY Stage Move Limit (µm)"=w799:dbl)
              n433 = Array Subset(array=w766, index (row)=0 ("index"), length (row)=2 ("length"), index (col)=3 ("index"), length (col)=1 ("length")) -> (w765:dbl[][])
              n434 = Index Array(array=w765, index (col)=0 ("disabled index (col)")) -> (element=w763:dbl[])  [unwired: 1 in]
              n435 = Equal?(x=4Pi_Obj_Lock_-_Actions."Move XYZ", y=w776) -> (x = y?=w774:bool)
              n436 = Build Array("X Update Scale Factor", "Y Update Scale Factor") -> (w757:dbl[])
              n437 = Select(t=4Pi_Obj_Lock_-_Actions."Move Z" ("x"), s=w774, f=4Pi_Obj_Lock_-_Actions."Update Plots") -> (s? t:f=w771:T6)
              n438 = Multiply(x=w761, y=w757) -> (x*y=w760:dbl[])
              n439 = call "Stages Messenger.vi"("Stage Notifier Name"=w780, "Actions"=Stage_Actions."Get Position") -> ("Stage Notifier Name (Dup)"=w779:string, "Positions"=w778:dbl[])  [unwired: 10 in, 2 out]
              n440 = call "4Pi Obj Lock - Rotate Flip XY.vi"("XY Amounts"=w760, "Flip XY"="Flip XY Axis", "Invert X"="Invert X Axis", "Invert Y"="Invert Y Axis") -> ("45° Rotated XY"=w762:dbl[])  [unwired: 11 in]
              n441 = Add(x=w778, y=w762) -> (x+y=w777:dbl[])
              n442 = Add(x=w763, y=w788) -> (x+y=w786:dbl[])
              n443 = Subtract(x=w763, y=w788) -> (x-y=w787:dbl[])
              n444 = Absolute Value(x=w762) -> (abs(x)=w798:dbl[])
              n445 = Greater?(x=w799, y=w798) -> (0:w797:bool[])
              n446 = In Range and Coerce(upper limit=w786, x=w777, lower limit=w787) -> (In Range?=w785:bool[])  [unwired: 1 out]
              n447 = And Array Elements(Boolean array=w797) -> (logical AND=w784:bool)
              n448 = And Array Elements(Boolean array=w785) -> (logical AND=w782:bool)
              n449 = And(x=w784, y=w782) -> (x .and. y?=w783:bool)
              n450 = Not(x=w783) -> (.not. x?=→"Move Limit Error":bool)
              n451 = case shown="True" w783 {
                tunnel: w762 -> [_ w823]
                tunnel: w796 -> [w819 _]
                tunnel: [w817 w820] -> w795
                tunnel: w779 -> [_ w822]
                tunnel: [dbl[] [-1.0, -1.0] ("Positions") w821] -> w793
                tunnel: w771 -> [w815 w820]
                frame False {
                  n452 = Select(t=4Pi_Obj_Lock_-_Actions."Abort" ("x"), s=w819, f=w815) -> (s? t:f=w817:T6)
                }
                frame True {
                  n453 = call "Stages Messenger.vi"("Stage Notifier Name"=w822, "Actions"=Stage_Actions."MVR", "Setpoint"=w823, "Axis"=bool[] [TRUE, TRUE]) -> ("Positions"=w821:dbl[])  [unwired: 8 in, 3 out]
                }
              }
              n454 = Index Array(array=w793, index #1=0 ("index"), index #2=1 ("index")) -> (element #1=→"X Axis Position (µm)":dbl, element #2=→"Y Axis Position (µm)":dbl)
            }
            frame "Move Z" {
              w839 = 2.0 ("y")
              # "Initial Z stage position"
              n455 = Get Notifier Status(notifier=w857) -> (notifier out=w856:refnum<notifier>, current notification=w858:T8)  [unwired: 1 in, 3 out]
              n456 = case shown="False" FALSE {
                tunnel: [w860 w863] -> w851
                tunnel: w833 -> [_ w861]
                frame False {
                  n457 = local read "dz (µm)"() -> (w860:dbl)
                }
                frame True {
                  w862 = 0 ("disabled index (col)")
                  # "Get sx/sy Diff Value"
                  n458 = Array Subset(array=w861, index (row)=2 ("index"), length (row)=1 ("length"), index (col)=2 ("index"), length (col)=1 ("length")) -> (w865:dbl[][])
                  n459 = Index Array(array=w865, index (row)=w862, index (col)=w862) -> (element=w863:dbl)
                }
              }
              n460 = Index Array(array=w833, index (row)=2, index (col)=3 ("disabled index (col)")) -> (element=w830:dbl)
              n461 = Unbundle By Name(w858) -> ("Abort If Error"=w838:bool, "Z Stage Move Limit (µm)"=w843:dbl)
              n462 = Multiply(x=w851, y="Z Update Scale Factor") -> (x*y=w848:dbl)
              n463 = Add(x=w830, y=w839) -> (x+y=w845:dbl)
              n464 = Subtract(x=w830, y=w839) -> (x-y=w844:dbl)
              n465 = call "Stages Messenger.vi"("Stage Notifier Name"=w854, "Actions"=Stage_Actions."Get Position") -> ("Stage Notifier Name (Dup)"=w840:string, "Positions"=w852:dbl[])  [unwired: 10 in, 2 out]
              n466 = Negate(x=w848) -> (-x=w849:dbl)
              n467 = Select(t=w849, s="Invert Z Axis", f=w848) -> (s? t:f=w829:dbl)
              n468 = Index Array(array=w852, index=0) -> (element=w850:dbl)
              n469 = Absolute Value(x=w829) -> (abs(x)=w828:dbl)
              n470 = Add(x=w829, y=w850) -> (x+y=w846:dbl)
              n471 = Greater?(x=w843, y=w828) -> (0:w842:bool)
              n472 = In Range and Coerce(upper limit=w845, x=w846, lower limit=w844) -> (In Range?=w841:bool)  [unwired: 1 out]
              n473 = And(x=w842, y=w841) -> (x .and. y?=w837:bool)
              n474 = Not(x=w837) -> (.not. x?=w836:bool)
              n475 = case shown="True" w837 {
                tunnel: w840 -> [_ w882]
                tunnel: w838 -> [w872 _]
                tunnel: w829 -> [_ w881]
                tunnel: [w871 4Pi_Obj_Lock_-_Actions."Update Plots" ("x")] -> w835
                tunnel: [-1.0 ("Position") w876] -> w834
                frame False {
                  n476 = Select(t=4Pi_Obj_Lock_-_Actions."Abort" ("x"), s=w872, f=4Pi_Obj_Lock_-_Actions."Update Plots") -> (s? t:f=w871:T6)
                }
                frame True {
                  n477 = Build Array(w881) -> (w880:dbl[])
                  n478 = call "Stages Messenger.vi"("Stage Notifier Name"=w882, "Actions"=Stage_Actions."MVR", "Setpoint"=w880, "Axis"=bool[] [TRUE]) -> ("Positions"=w878:dbl[])  [unwired: 8 in, 3 out]
                  n479 = Wait (ms)(milliseconds to wait=u32 50) -> ()  [unwired: 1 out]
                  n480 = Index Array(array=w878, index=0) -> (element=w876:dbl)
                }
              }
              "Z Axis Position (µm)" <- w834
              n481 = local write "Move Limit Error"(w836) -> ()
            }
            frame "Update Plots" {
              # "Current Values"
              # "Target Values"
              n482 = Get Notifier Status(notifier=w937) -> (notifier out=w936:refnum<notifier>, current notification=w938:T8)  [unwired: 1 in, 3 out]
              n483 = Unbundle By Name(w938) -> ("Z Drift Threshold"=w928:dbl, "XY Drift Threshold"=w927:dbl)
              n484 = local read "X Axis Position (µm)"() -> (w922:dbl)
              n485 = local read "Y Axis Position (µm)"() -> (w921:dbl)
              n486 = local read "Z Axis Position (µm)"() -> (w920:dbl)
              n487 = Index Array(array=w917, index (col)=0 ("disabled index (col)")) -> (element=w912:dbl[])  [unwired: 1 in]
              n488 = Index Array(array=w917, index (col)=1 ("disabled index (col)")) -> (element=w913:dbl[])  [unwired: 1 in]
              n489 = Index Array(array=w917, index (col)=3 ("disabled index (col)")) -> (element=w918:dbl[])  [unwired: 1 in]
              n490 = Subtract(x=w913, y=w912) -> (x-y=w911:dbl[])
              n491 = local read "Measured X Position cc (px)"() -> (w897:dbl)
              n492 = local read "Measured Y Position cc (px)"() -> (w896:dbl)
              n493 = local read "Target Y Position cc (px)"() -> (w898:dbl)
              n494 = Build Array(w922, w921, w920) -> (w919:dbl[])
              n495 = local read "Target X Position cc (px)"() -> (w899:dbl)
              n496 = Index Array(array=w911, index #1=0 ("index"), index #2=1 ("index"), index #3=2 ("index")) -> (element #1=w895:dbl, element #2=w894:dbl, element #3=w903:dbl)
              n497 = Subtract(x=w919, y=w918) -> (x-y=w916:dbl[])
              n498 = Build Array(w895, w894) -> (w892:dbl[])
              n499 = Index Array(array=w916, index #1=0 ("index"), index #2=1 ("index"), index #3=2 ("index")) -> (element #1=w915:dbl, element #2=w914:dbl, element #3=w902:dbl)
              n500 = Build Array(w896, w897) -> (w900:dbl[])
              n501 = Build Array(w898, w899) -> (w901:dbl[])
              n502 = Subtract(x=w900, y=w901) -> (x-y=w893:dbl[])
              n503 = Select(t=w892, s=FALSE, f=w893) -> (s? t:f=w890:dbl[])
              n504 = Multiply(x="pixel size (µm)", y=w890) -> (x*y=w888:dbl[])
              n505 = Index Array(array=w888, index #1=0 ("index"), index #2=1 ("index")) -> (element #1=w885:dbl, element #2=w884:dbl)
              n506 = call "4Pi Obj Lock - 1 Values Organize Plot Data.vi"("Target 01"=0.0, "Value Limit"=w927, "Current 01"=w885, "Stage Pos"=w915) -> ("plot data"=→"X Target and Fit Position (µm)":T2)  [unwired: 11 in]
              n507 = call "4Pi Obj Lock - 1 Values Organize Plot Data.vi"("Target 01"=0.0, "Value Limit"=w927, "Current 01"=w884, "Stage Pos"=w914) -> ("plot data"=→"Y Target and Fit Position (µm)":T2)  [unwired: 11 in]
              n508 = local read "Measured Z (µm)"() -> (w906:dbl)
              n509 = Select(t=w903, s=FALSE, f=w906) -> (s? t:f=w904:dbl)
              n510 = call "4Pi Obj Lock - 1 Values Organize Plot Data.vi"("Target 01"=0.0, "Value Limit"=w928, "Current 01"=w904, "Stage Pos"=w902) -> ("plot data"=→"Z Target and Fit Value (µm)":T2)  [unwired: 11 in]
            }
            frame "Delay" {
              n511 = Get Notifier Status(notifier=w946) -> (notifier out=w944:refnum<notifier>, current notification=w947:T8)  [unwired: 1 in, 3 out]
              n512 = Unbundle By Name(w947) -> ("Update Delay (ms)"=w943:i32)
              n513 = while {
                tunnel: w944 -> [w959]
                tunnel: w943 -> [w956]
                tunnel: [w952] -> w942
                i -> [w957]
                stop <- w950 stop-if-true
                n514 = Get Notifier Status(notifier=w959) -> (notifier out=w952:refnum<notifier>, current notification=w955:T8)  [unwired: 1 in, 3 out]
                n515 = Greater Or Equal?(x=w957, y=w956) -> (x >= y?=w951:bool)
                n516 = Wait (ms)(milliseconds to wait=u32 1) -> ()  [unwired: 1 out]
                n517 = Unbundle By Name(w955) -> ("Actions"=w954:T6)
                n518 = Equal?(x=w954, y=4Pi_Obj_Lock_-_Actions."Abort") -> (x = y?=w949:bool)
                n519 = Or(x=w949, y=w951) -> (x .or. y?=w950:bool)
              }
            }
            frame "Abort" {
              w963 = 0.0 ("Target X Position (px)")
              n520 = Get Notifier Status(notifier=w969) -> (notifier out=w973:refnum<notifier>, current notification=w972:T8)  [unwired: 1 in, 3 out]
              n521 = call "Camera Messenger.vi"("Notifier Name"=w961, "General Camera Actions"=Generic_Camera_Actions."Abort") -> ()  [unwired: 8 in, 6 out]
              n522 = Bundle By Name(cluster=w972, "Running?"=FALSE, "Actions"=4Pi_Obj_Lock_-_Actions."Exit Loop") -> (w970:T8)
              n523 = Send Notification(notification=w970, notifier=w973) -> (notifier out=w968:refnum<notifier>)  [unwired: 1 in, 1 out]
              n524 = local write "Start Lock"(FALSE ("Start Lock")) -> ()
              n525 = local write "Measured X Position (px)"(w963) -> ()
              n526 = local write "Measured Y Position (px)"(w963) -> ()
              n527 = local write "Target X Position (px)"(w963) -> ()
              n528 = local write "Target Y Position (px)"(w963) -> ()
              n529 = local write "Measured sx/sy"(w963) -> ()
              n530 = local write "Target sx/sy"(w963) -> ()
            }
            frame "Exit Loop" {
            }
            frame "Quit" {
              n531 = Get Notifier Status(notifier=w979) -> (notifier out=w978:refnum<notifier>, current notification=w986:T8)  [unwired: 1 in, 3 out]
              n532 = Unbundle By Name(w986) -> ("Ref Stack (SGL)"=w985:T9[], "Cur Image (SGL)"=w984:T9, "Tmp Image FFT (CSG)"=w983:T9[], "CC Image (SGL)"=w982:T9, "Ref FFT Stack (CSG)"=w980:T9[])
              n533 = Release Notifier(notifier=w978, force destroy? (F)=TRUE) -> ()  [unwired: 1 in, 3 out]
              n534 = Build Array (concatenate)(w985, w984, w983, w982, w980) -> (w981:T9[])
              n535 = for {
                tunnel: w981 -> [w991] mode=indexing
                n536 = call "IMAQ Dispose"("Image"=w991) -> ()  [unwired: 5 in, 1 out]
              }
            }
          }
          n537 = Get Notifier Status(notifier=w234) -> (current notification=w233:T8, error out=w228:errorcluster)  [unwired: 1 in, 3 out]
          n538 = Unbundle By Name(w233) -> ("Actions"=w232:T6)
          n539 = Unbundle By Name(w228) -> ("status"=w226:bool)
          n540 = Equal?(x=w231, y=w232) -> (x = y?=w227:bool)
          n541 = Or(x=w227, y=w226) -> (x .or. y?=w225:bool)
          n542 = Select(t=w231, s=w225, f=w230) -> (s? t:f=w229:T6)
        }
      }
      n543 = local write "Quit"(w208) -> ()
    }
    frame Error {
    }
  }
  n544 = control-ref of="This VI"() -> (w87:refnum<vi>)
  n545 = property class="VI"(reference=w87) -> (reference out=w96:refnum<vi>, "Panel"=w88:refnum<vi>)  [unwired: 1 in, 1 out]
  n546 = property class="Pnl"(reference=w88) -> ("Decos[]"=w86:refnum<vi>[], "Panes[]"=w92:refnum<vi>[])  [unwired: 1 in, 2 out]
  n547 = Array Size(array=w86) -> (size(s)=w84:i32)
  n548 = Decrement(x=w84) -> (x-1=w85:i32)
  n549 = Index Array(array=w92, index=0) -> (element=w91:refnum<vi>)
  n550 = Index Array(array=w86, index=w85) -> (element=w94:refnum<vi>)
  n551 = property class="VI"(reference=w96) -> (reference out=w98:refnum<vi>, "Front Panel.PanelBounds"=w99:T22)  [unwired: 1 in, 1 out]
  n552 = property class="Decor"(reference=w94) -> ("Bounds"=w97:T23)  [unwired: 1 in, 2 out]
  n553 = property class="Pane"(reference=w91, "Origin"=T11 {"Horizontal"=0, "Vertical"=0}, "HorizScrollbarVisibility"=w95, "VertScrollbarVisibility"=w95) -> ()  [unwired: 1 in, 2 out]
  n554 = Unbundle By Name(w97) -> ("Width"=w102:u32, "Height"=w105:u32)
  n555 = control-ref of="Quit"() -> (w89:refnum<vi>)
  n556 = To Word Integer(number=w102) -> (16bit integer=w104:i16)
  n557 = To Word Integer(number=w105) -> ()  [unwired: 1 out]
  n558 = property class="Bool (strict)"(reference=w89) -> ("Height"=w107:u32, "Top"=w108:i32)  [unwired: 1 in, 2 out]
  n559 = Unbundle By Name(w99) -> ("Left"=w101:i16, "Top"=w112:i16)
  n560 = To Word Integer(number=w107) -> (16bit integer=w110:i16)
  n561 = To Word Integer(number=w108) -> (16bit integer=w111:i16)
  n562 = Add(x=w101, y=w104) -> (x+y=w103:i16)
  n563 = Compound Arithmetic op=ADD(w112, w110, w111, i16 12 ("y")) -> (w106:i16)
  n564 = Bundle By Name(cluster=w99, "Right"=w103, "Bottom"=w106) -> (w100:T22)
  n565 = property class="VI"(reference=w98, "Front Panel.PanelBounds"=w100) -> ()  [unwired: 1 in, 2 out]
